vi "Test Executive.vi"(11 "Module Config":T3={"Name"="TestExec", "Parent Q"=refnum, "Is Child?"=FALSE, "Index"=0, "Dirs"={"Root"=path "", "Config"=path "C:/ATE/Config", "Logs"=path "C:/ATE/Logs", "Reports"=path "C:/ATE/Reports", "App Data"=path "C:/ProgramData/MAIN"}, "Simulate"=FALSE}) -> ()   [LabVIEW 2017]
uses:
  <vilib>/KATE/Queues/Queue Utils.lvlib
  <vilib>/KATE/Module/Module Utils.lvlib
  <vilib>/KATE/Module/Window/Window.Task, Action.ctl
  <vilib>/KATE/Event Log/Event Log.lvlib
  <vilib>/KATE/Scheduler/Scheduler.lvlib
  <vilib>/KATE/Files/File Utils.lvlib
  <vilib>/KATE/Menu/Menu Utils.lvlib
  <vilib>/KATE/Event Log/Event Log.Error Report.ctl
  <vilib>/KATE/Controls/Controls.lvlib
  Controls/TestExec.TestState.ctl
  <vilib>/KATE/Queues/Q.Element.ctl
  <vilib>/KATE/Queues/Q.Msg Return Info.ctl
  <vilib>/KATE/Queues/Q.Msg Return Data Container.ctl
  Controls/TestExec.Script Message.ctl
  <vilib>/Utility/miscctls.llb/LVRowAndColumnUnsignedTypeDef.ctl
  SubVIs/Class - ResultCntr/Class - ResultCntr.lvclass
  <vilib>/KATE/Graphics/Graphic Utils.lvlib
  <vilib>/KATE/Config/Stored Controls/Class.SaveCtrls.lvclass
  Common/TCP-IP Manager/TCP-IP Mgr.lvlib
  <vilib>/KATE/Module/Module Config.ctl
  <vilib>/KATE/Module/Module.Working Dirs.ctl
  <vilib>/KATE/Module/Module.SW Version Info.ctl
panel:
  in  "Main Tab":enum32{"Operate", "Maint"}(tab)
  out "Facility Name":string caption="Name"
  out "Error":bool
  out "Error":bool
  out "Title":string="Test Executive"
  in  "Data Tab":T1(tab)
  out "Rev":string
  in  "Sequence":u16(ring) items=["Test AAA 001", "Test BBB 002", "Test CCC 003"]
  out "Test Status Tab":enum32{"Results", "Setup"}(tab)
  out "Results":string[][](table)
  out "Setup/Instuction Figure":picture
  out "Data2DBool":bool[][](array[boolean])=[[TRUE, FALSE], [FALSE, TRUE]]
  out "Data2DStr":string[][](array[string])=[["A", "AA"], ["B", "BB"], ["C", "CC"], ["D", "DD"]]
  out "UUT State":T2={"Standby"=TRUE, "Initializing"=FALSE, "Running"=FALSE, "Error"=FALSE}
  out "Data2DFloat":dbl[][](array[numeric])
  out "Data1DFloat":dbl[](array[numeric])
  in  "ON/OFF":bool
  out "OutputY":dbl
  out "OutputX":dbl
  out "Data1DBool":bool[](array[boolean])=[TRUE, TRUE, FALSE, TRUE]
  out "Output Hist":cluster{dbl, dbl}(graph)
  in  "Equipment List":string[][](table)=[["Function Generator", "", "", "", ""], ["", "", "", "", ""], ["", "", "", "", ""], ["", "", "", "", ""], ["", "", "", "", ""]]
  out "Status":string
  out "Test Ctrl Tab":enum32{"Idle", "Running", "Completed"}(tab)
  in  "Start":bool
  out "Status Duration(s)":dbl caption="Duration(s)" format="%.1f"
  out "Status Elapsed(s)":dbl caption="Elapsed(s)" format="%.1f"
  out "Test Running":bool
  out "Progress":dbl(slide) scale=0.0..1.0
  in  "Abort":bool
  in  "Test Reset":bool
  out "Operator":string
  out "Station PN":string caption="PN"
  out "Station SN":string caption="SN"
  in  "UUT PN":string caption="PN"
  in  "UUT SN":string caption="SN"
  out "Start Time":string
  out "End Time":string
  in  "Maint":bool
  out "Logo":picture
  in  "Show Block Diagram":bool
  in  "Leave Maint":bool
  in  "SW Rev":T5={"AppName"="Test Executive", "Company"="Kwest Engineering", "Version"="0.0.3", "Description"="4/8/2017"}
  # "Facility"
  # "Station"
  # "UUT"
  # "There is a 2 sec delay from turn ON\nto Running sTATE"
  # "0"
  # "1"
  # "2"
  # "3"
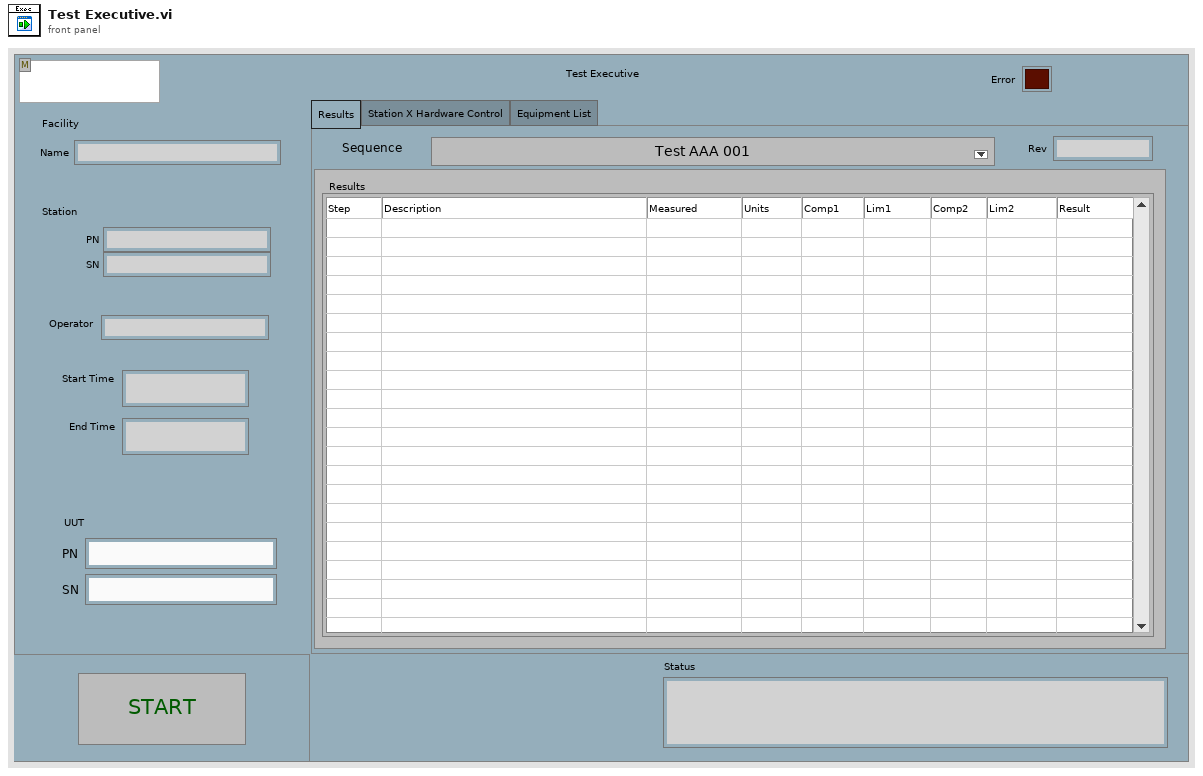
[diagram p1: front panel]
types:
  T1 = enum32{"Results", "Station X Hardware Control", "Equipment List"}
  T2 = cluster{"Standby":bool, "Initializing":bool, "Running":bool, "Error":bool}
  T3 = typedef "KATE_Lib.lvlib/Module Utils.lvlib/Module Config.ctl" = cluster{"Name":string, "Parent Q":refnum<queue>, "Is Child?":bool, "Index":i32, "Dirs":T4, "Simulate":bool}
  T4 = typedef "KATE_Lib.lvlib/Module Utils.lvlib/Module.Working Dirs.ctl" = cluster{"Root":path, "Config":path, "Logs":path, "Reports":path, "App Data":path}
  T5 = typedef "KATE_Lib.lvlib/Module Utils.lvlib/Module.SW Version Info.ctl" = cluster{"AppName":string, "Company":string, "Version":string, "Description":string}
  T6 = typedef "KATE_Lib.lvlib/Module Utils.lvlib/Module Sys Info.ctl" = cluster{"Main Q":refnum<queue>, "Exe":bool, "SW Rev":T5, "Self Ref":refnum<vi>, "Main Tab":refnum<vi>, "Pane":refnum<vi>, "Stop":cluster{"Ref":refnum<event-registration>, "Event":refnum<user-event>}, "Cfg":T3, "Services":cluster{"Name":string, "vi ref":refnum<vi>}[], "Menu Ref":refnum<k9>, "CtrlStates":refnum<class "Class.SaveCtrls.lvclass">, "Docs":cluster{"Tags":string[], "Paths":path[]}}
  T7 = enum8{"Enabled", "Disabled", "Disabled and Grayed Out"}
  T8 = typedef "LVRowAndColumnUnsignedTypeDef.ctl" = cluster{"Row":u32, "Column":u32}
  T9 = typedef "TestExec.TestState.ctl" = cluster{"Running":bool, "Results":string[][], "Start":dbl, "End":dbl, "Duration":dbl, "Failing":bool, "Abort":bool, "TC Level":i32, "TC Cnts":i32[], "Test ID":string}
  T10 = typedef "TestExec.Script Message.ctl" = cluster{"Seq":i32, "Address":string, "Function":string, "Data":variant, "Error":errorcluster}
  T11 = typedef "KATE_Lib.lvlib/Queue Utils.lvlib/Q.Msg Return Data Container.ctl" = cluster{"SeqNum":i32, "Data":variant, "Error":errorcluster}
  T12 = enum16{"Top Left", "Top Right", "Bottom Left", "Bottom Right"}
  T13 = cluster{"CtrlStates":refnum<class "Class.SaveCtrls.lvclass">, "Test":T9, "Limits":variant, "ResultID":refnum<class "Class - ResultCntr.lvclass">}
  T14 = typedef "KATE_Lib.lvlib/Queue Utils.lvlib/Q.Msg Return Info.ctl" = cluster{"Ret Q":refnum<queue>, "Ret Msg":T15, "SeqNum":i32}
  T15 = typedef "KATE_Lib.lvlib/Queue Utils.lvlib/Q.Element.ctl" = cluster{"Cmd":string, "Sub":string, "Data1":variant, "Data2":variant}
  T16 = typedef "KATE_Lib.lvlib/Event Log.lvlib/Event Log.Error Report.ctl" = cluster{"Cnt":i32, "Recent Error":errorcluster}
  T17 = typedef "KATE_Lib.lvlib/Module Utils.lvlib/Window.Task, Action.ctl" = enum16{"Resize()", "Show Panel(Bool)", "Show Scroll Bars(Bool)", "Dock to SubPanel(SubPanel Ref)", "Undock from SubPanel()", "Return to SubPanel()", "Go To Maint Tab()", "Show Maint Tab(Bool)", "Open Block Diagram()"}
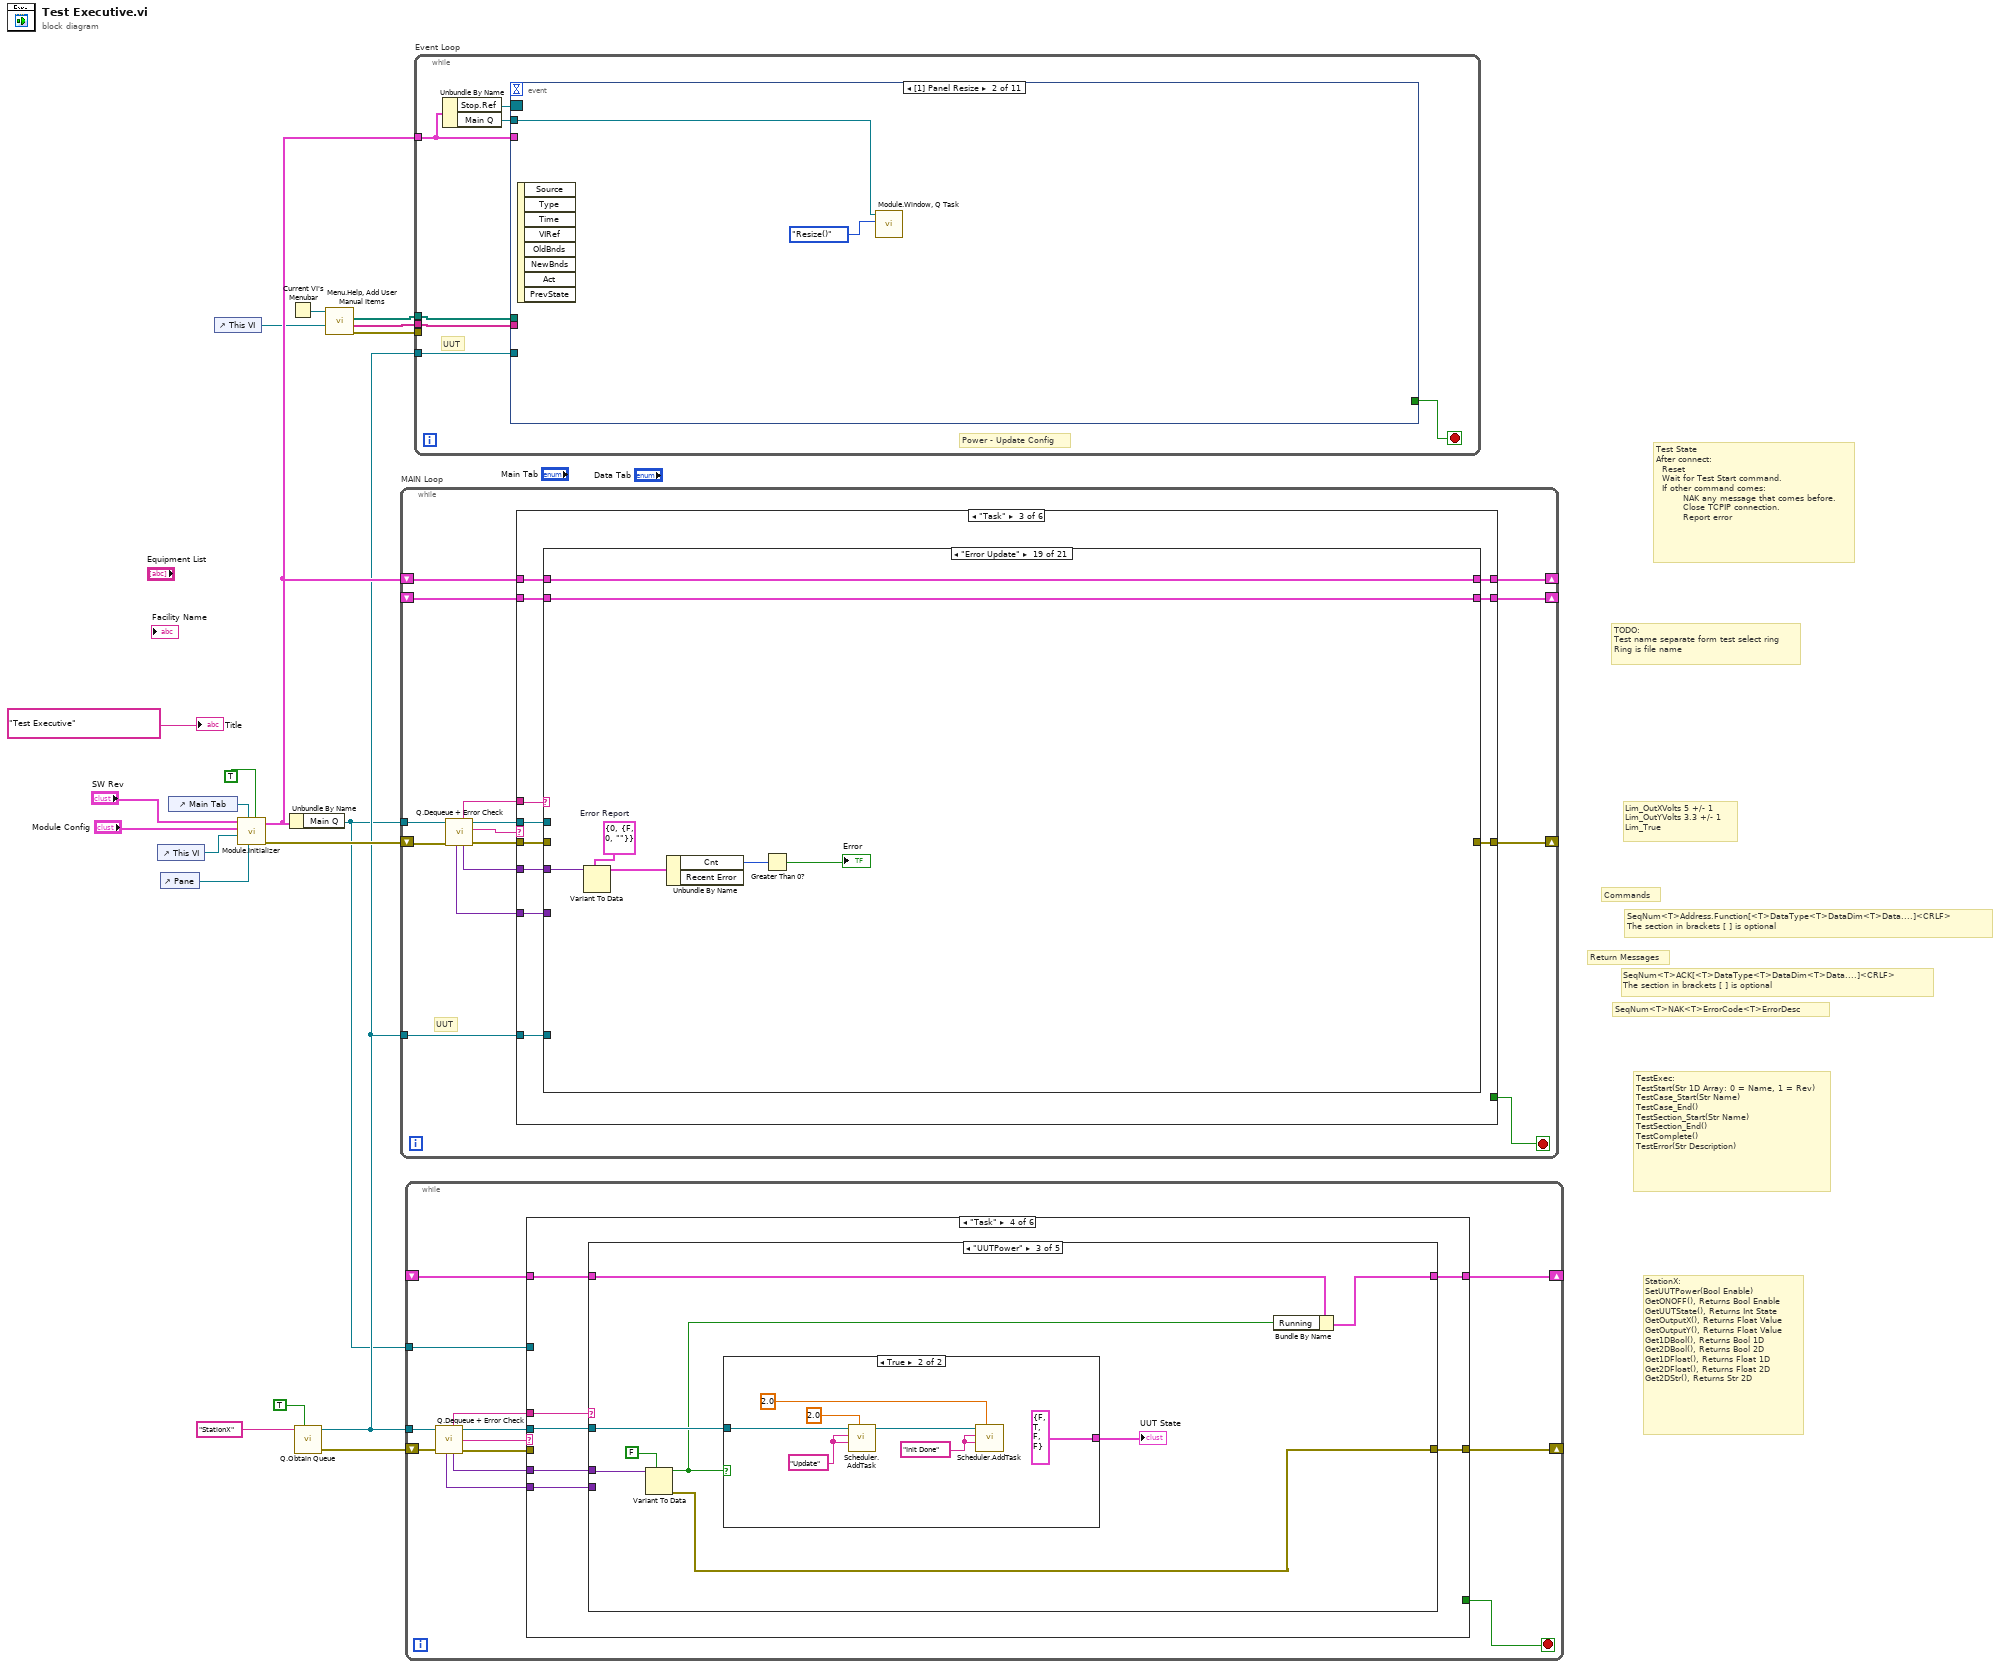
[diagram p0: block diagram]
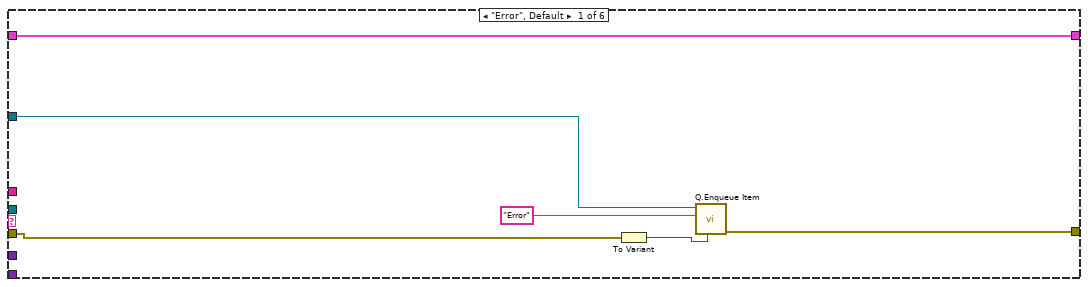
[diagram p2: hidden frame]
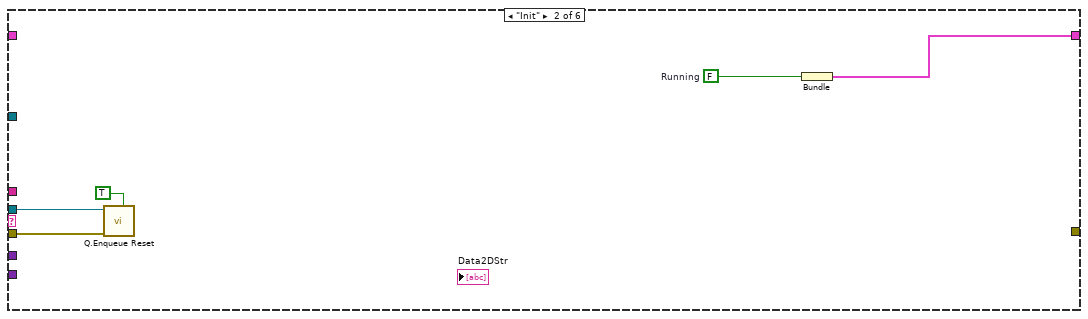
[diagram p3: hidden frame]
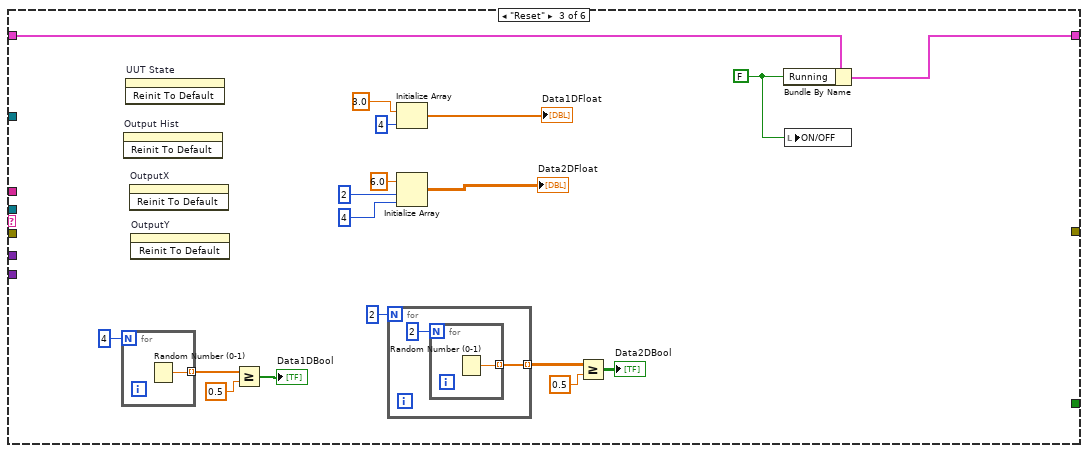
[diagram p4: hidden frame]
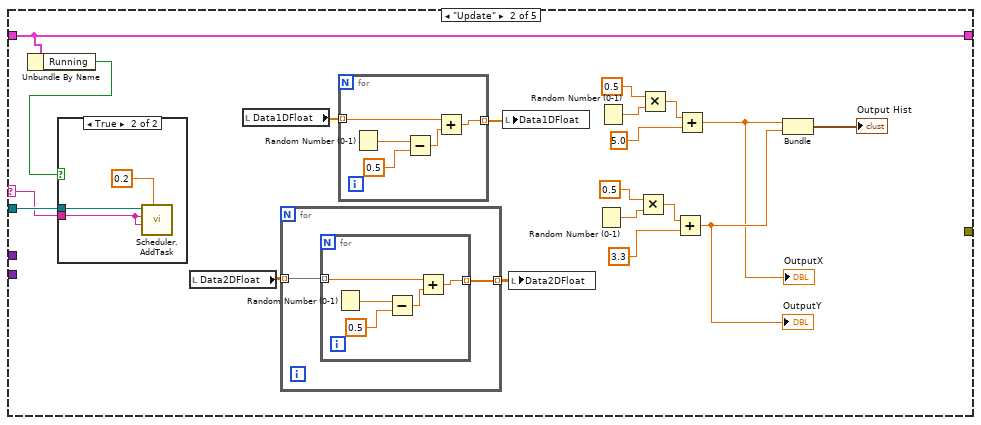
[diagram p6: hidden frame]
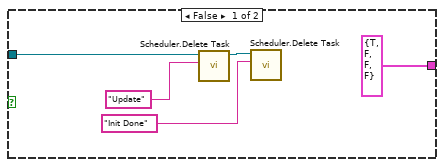
[diagram p8: hidden frame]
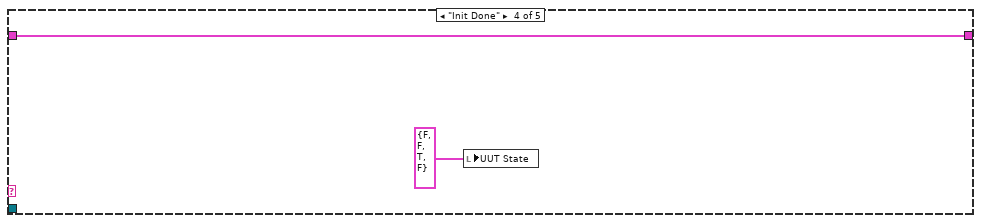
[diagram p9: hidden frame]
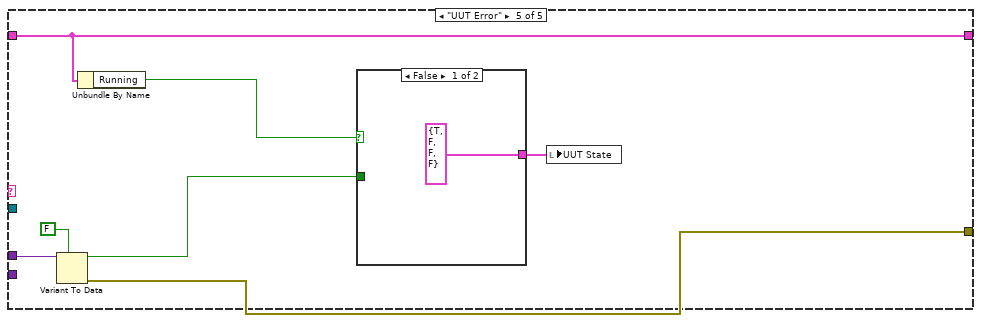
[diagram p10: hidden frame]
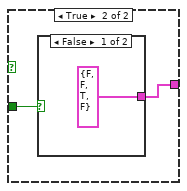
[diagram p11: hidden frame]
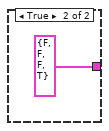
[diagram p12: hidden frame]
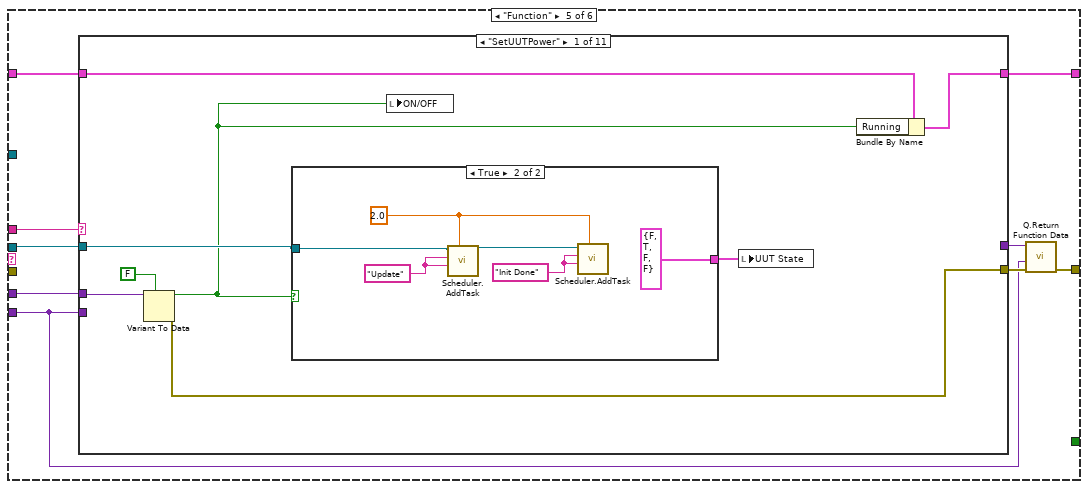
[diagram p13: hidden frame]
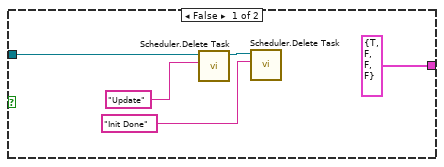
[diagram p14: hidden frame]
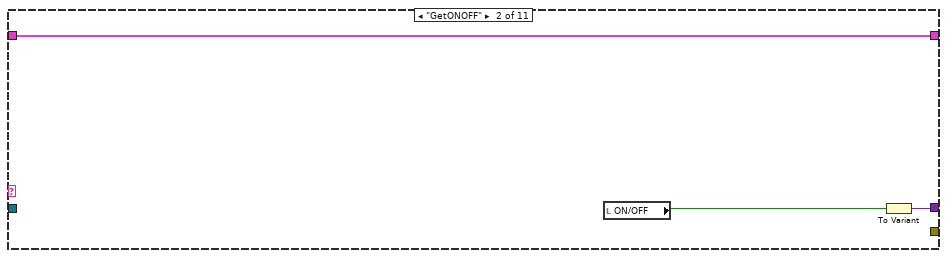
[diagram p15: hidden frame]
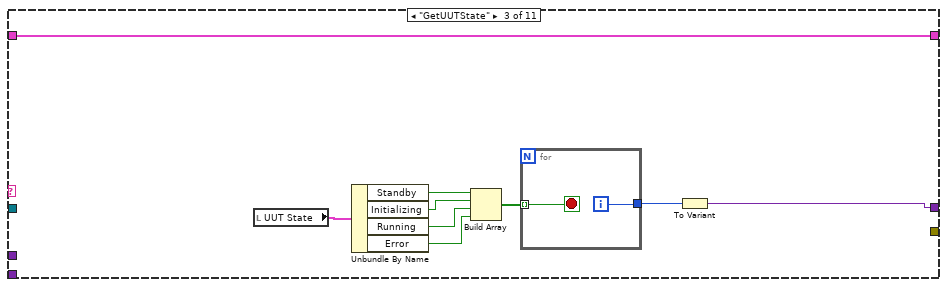
[diagram p16: hidden frame]
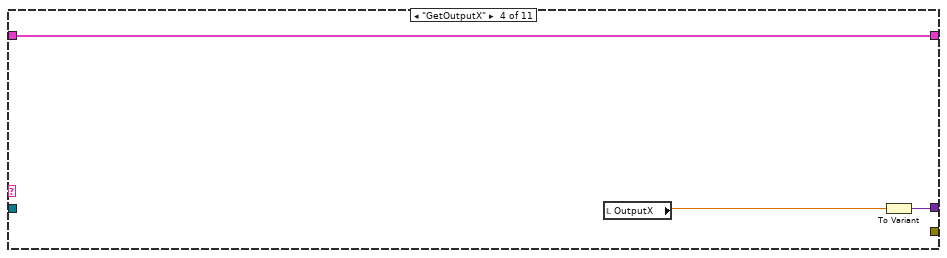
[diagram p17: hidden frame]
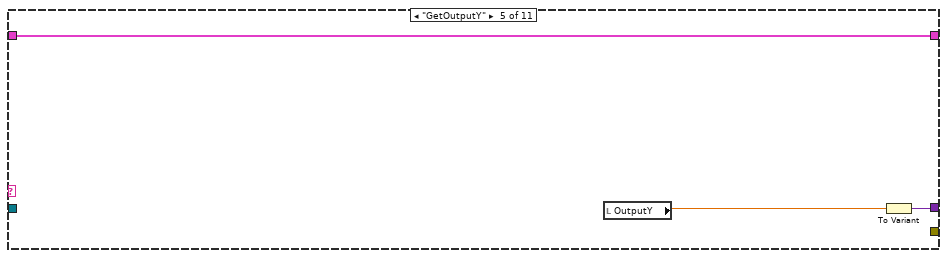
[diagram p18: hidden frame]
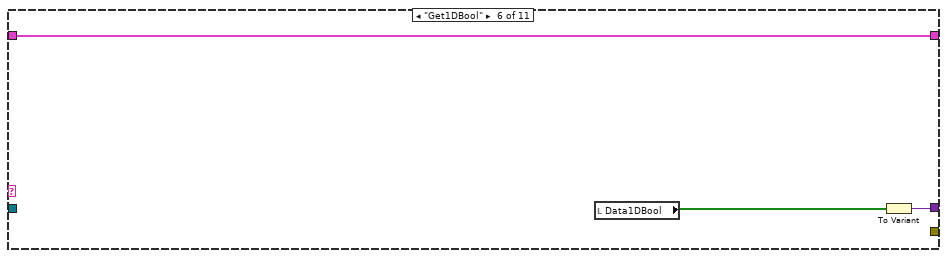
[diagram p19: hidden frame]
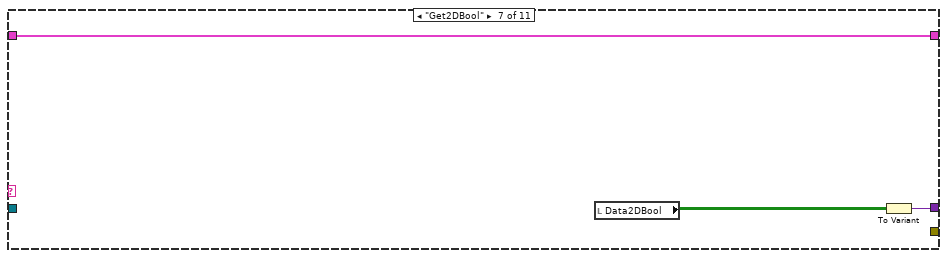
[diagram p20: hidden frame]
diagram:
  # "TODO:\nTest name separate form test select ring\nRing is file name"
  # "Test State\nAfter connect:\n  Reset\n  Wait for Test Start command.\n  If other command comes: \n         NAK any message that comes before.\n         Close TCPIP connection.\n         Report error"
  # "Lim_OutXVolts 5 +/- 1\nLim_OutYVolts 3.3 +/- 1\nLim_True"
  # "Return Messages"
  # "Commands"
  # "SeqNum<T>NAK<T>ErrorCode<T>ErrorDesc"
  # "SeqNum<T>ACK[<T>DataType<T>DataDim<T>Data....]<CRLF>  \nThe section in brackets [ ] is optional"
  # "SeqNum<T>Address.Function[<T>DataType<T>DataDim<T>Data....]<CRLF>\nThe section in brackets [ ] is optional"
  # "StationX:\nSetUUTPower(Bool Enable)\nGetONOFF(), Returns Bool Enable\nGetUUTState(), Returns Int State\nGetOutputX(), Returns Float Value\nGetOutputY(), Returns Float Value\nGet1DBool(), Returns Bool 1D\nGet2DBool(), Returns Bool 2D\nGet1DFloat(), Returns Float 1D\nGet2DFloat(), Returns Float 2D\nGet2DStr(), Returns Str 2D"
  # "TestExec:\nTestStart(Str 1D Array: 0 = Name, 1 = Rev)\nTestCase_Start(Str Name)\nTestCase_End()\nTestSection_Start(Str Name)\nTestSection_End()\nTestComplete()\nTestError(Str Description)"
  n1 = control-ref of="This VI"() -> (w17:refnum<vi>)
  n2 = control-ref of="Pane"() -> (w16:refnum<vi>)
  n3 = control-ref of="Main Tab"() -> (w18:refnum<vi>)
  n4 = control-ref of="This VI"() -> (w3:refnum<vi>)
  n5 = call <vilib>:"Module.Initializer.vi"("Menu Ref"=TRUE ("En Event Log"), "Pane"=w16, "Main Tab"=w18, "Self Ref"=w17, "Module Config"="Module Config", "SW Rev"="SW Rev") -> ("error out"=w19:errorcluster, "Sys"=w9:T6)  [unwired: 4 in]
  n6 = Current VI's Menubar() -> (w13:refnum<k9>)
  n7 = Unbundle By Name(w9) -> ("Main Q"=w4:refnum<queue>)
  n8 = call <vilib>:"Q.Obtain Queue.vi"("Enqueue Init"=TRUE, "Q Name"="StationX" ("Name")) -> ("error out"=w8:errorcluster, "Q Out"=w5:refnum<queue>)  [unwired: 7 in, 1 out]
  n9 = call <vilib>:"Menu.Help, Add User Manual Items.vi"("Main VI"=w3, "Menu Ref"=w13) -> ("error out"=w12:errorcluster, "Tags"=w11:string[], "Paths"=w10:path[])  [unwired: 6 in, 1 out]
  n10 = while "MAIN Loop" {
    shift-right: [w30] -> _
    shift-left: w19 -> [w28]
    shift-right: [w31] -> _
    shift-left: _ -> [w34]
    shift-right: [w32] -> _
    shift-left: w9 -> [w33]
    tunnel: w4 -> [w27]
    tunnel: w5 -> [w20]
    stop <- w21 stop-if-true
    # "UUT"
    n11 = call <vilib>:"Q.Dequeue + Error Check.vi"("Error In"=w28, "Q In"=w27) -> ("error out"=w29:errorcluster, "Cmd"=w26:string, "Q Out"=w25:refnum<queue>, "Data1"=w24:variant, "Sub"=w22:string, "Data2"=w23:variant)  [unwired: 4 in]
    n12 = case shown="\"Task\"" w26 {
      selector: w26 -> [_ _ _ _ w668 _]
      tunnel: w34 -> [_ w87 w135 w531 w662 w715]
      tunnel: w33 -> [w42 w117 w136 w532 w670 w716]
      tunnel: [w42 w117 w134 w530 w670 w716] -> w32
      tunnel: [w39 w120 w133 w529 w661 w715] -> w31
      tunnel: [w36 _ w127 w524 w669 w718] -> w30
      tunnel: w29 -> [w44 w124 w129 w525 w666 _]
      tunnel: w25 -> [w45 w125 w130 w526 w664 _]
      tunnel: w24 -> [_ _ w131 w527 w667 _]
      tunnel: w23 -> [_ _ w128 w523 _ _]
      tunnel: w22 -> [_ _ w132 w528 w665 _]
      tunnel: [_ _ _ _ _ TRUE] -> w21
      tunnel: w20 -> [_ _ w126 _ _ w712]
      frame "Init" {
        n13 = call <vilib>:"Q.Enqueue Reset.vi"("Top of Q(T)"=FALSE ("Flush Q"), "Error In"=w44, "Q In"=w45) -> ("Q Out"=w35:refnum<queue>)  [unwired: 7 in, 1 out]
        n14 = stacked-sequence {
          tunnel: w42 -> [w49 w61 _ w83]
          tunnel: [_ w62 _ _] -> w41
          tunnel: [_ _ w79 _] -> w40
          tunnel: [_ _ w78 _] -> w38
          tunnel: [_ _ w77 _] -> w37
          tunnel: w35 -> [_ _ _ w84]
          tunnel: [_ _ _ w80] -> w36
          frame #0 {
            # "Only allow \"Show block diagram\" in development"
            n15 = call <vilib>:"Application Directory.vi"() -> ("Application Directory"=w48:path)
            n16 = Unbundle By Name(w49) -> ()  [unwired: 1 out]
            n17 = Build Path(base path=w48, name or relative path="Company Logo.png") -> (appended path=w46:path)
            n18 = Unbundle By Name(w49) -> ("Exe"=w56:bool)
            n19 = call <vilib>:"Image File to 2D Image.vi"("Path"=w46) -> ("2D Picture"=→"Logo":picture)  [unwired: 9 in, 1 out]
            n20 = Not(x=w56) -> (.not. x?=w57:bool)
            n21 = property on="Show Block Diagram" class="Bool"("Visible"=w57) -> ()  [unwired: 2 in, 2 out]
            n22 = property class="App"() -> ("App.UserName"=→"Operator":string)  [unwired: 2 in, 2 out]
            n23 = call <vilib>:"Event Log.Record Event.vi"("Message"="Application Launched") -> ()  [unwired: 10 in, 1 out]
            "Test Status Tab" <- enum32{"Results", "Setup"}."Results" ("Test Status Tab")
            "Station PN" <- "TS1034" ("Station PN")
            "Station SN" <- "001" ("Station PN")
          }
          frame #1 {
            (unwired) refnum<vi>[] []
            # "Restore saved control states"
            n24 = Unbundle By Name(w61) -> ("Cfg.Name"=w60:string, "Cfg.Dirs.App Data"=w59:path)
            n25 = while {
              shift-right: [w65] -> w58
              shift-left: _ -> [w66]
              i -> [w67]
              stop <- w64 stop-if-true
              n26 = case shown="0" w67 {
                tunnel: w66 -> [w69 w75]
                tunnel: [w69 w76] -> w65
                tunnel: [TRUE _] -> w64
                frame Default {
                  # "Done"
                }
                frame 0 {
                  w71 = refnum<vi> refnum  # Control
                  n27 = control-ref of="Sequence"() -> (w73:refnum<vi>)
                  n28 = control-ref of="Equipment List"() -> (w72:refnum<vi>)
                  n29 = To More Generic Class(target class=w71, reference=w73) -> (generic class reference=w74:refnum<vi>)
                  n30 = To More Generic Class(target class=w71, reference=w72) -> (generic class reference=w70:refnum<vi>)
                  n31 = Build Array (concatenate)(w75, w74, w70) -> (w76:refnum<vi>[])
                }
              }
            }
            n32 = call-dynamic "Class.SaveCtrls.InitLoadRestore.vi"("Ctrl Array"=w58, "Module Data Dir"=w59, "Module Name"=w60, "CtrlStates In"=refnum<class "Class.SaveCtrls.lvclass"> refnum) -> ("CtrlStates"=w62:refnum<class "Class.SaveCtrls.lvclass">)  [unwired: 6 in, 1 out]
          }
          frame #2 {
            w77 = refnum<class "Class - ResultCntr.lvclass"> refnum  # ResultID
            w78 = variant  # Limits
            w79 = T9 {"Running"=FALSE, "Results"=[], "Start"=0.0, "End"=0.0, "Duration"=0.0, "Failing"=FALSE, "Abort"=FALSE, "TC Level"=0, "TC Cnts"=[], "Test ID"=""}  # Test
          }
          frame #3 {
            # "Launch TCP-IP Listener"
            n33 = Unbundle By Name(w83) -> ("Cfg.Dirs"=w82:T4)
            n34 = call "TCP-IP Mgr.Create.vi"("Working Dirs"=w82, "Q In"=w84) -> ("Error Out"=w81:errorcluster)  [unwired: 7 in, 2 out]
            n35 = call "TCP-IP Mgr.Show.vi"("error in"=w81) -> ("error out"=w80:errorcluster)  [unwired: 10 in]
          }
        }
        n36 = Bundle("CtrlStates"=w41, "Test"=w40, "Limits"=w38, "ResultID"=w37) -> (w39:T13)  [unwired: 1 in]
      }
      frame "Reset" {
        w91 = FALSE ("Error")
        w105 = 0.0 ("Elapsed(s)")
        w107 = T9 {"Running"=FALSE, "Results"=[], "Start"=0.0, "End"=0.0, "Duration"=0.0, "Failing"=FALSE, "Abort"=FALSE, "TC Level"=0, "TC Cnts"=[], "Test ID"=""}  # Test
        w121 = 0
        n37 = call <vilib>:"Scheduler.Clear-Reset.vi"("error in"=w124, "Q In"=w125) -> ("error out"=w108:errorcluster, "Q Out"=w109:refnum<queue>)  [unwired: 8 in]
        n38 = Current VI's Menubar() -> (w112:refnum<k9>)
        n39 = property on="Error" class="Bool (strict)"("Visible"=FALSE) -> ()  [unwired: 2 in, 2 out]
        n40 = invoke on="Progress" class="Slide (strict)" method="Reinit To Default"() -> ()  [unwired: 3 in, 3 out]
        n41 = call <vilib>:"Menu.Enable Item.vi"("Enable"=TRUE, "Tag"="Config", "Menu Ref"=w112) -> ()  [unwired: 7 in, 2 out]
        n42 = invoke on="Error" class="Bool (strict)" method="Reinit To Default"() -> ()  [unwired: 3 in, 3 out]
        n43 = To Variant(anything=FALSE) -> (Variant=w115:variant)
        n44 = property on="Sequence" class="Ring (strict)"("Strings []"=string[] ["Test AAA 001", "Test BBB 002", "Test CCC 003"]) -> ()  [unwired: 2 in, 2 out]
        n45 = call <vilib>:"Q.Enqueue Task.vi"("Data1"=w115, "Error In"=w108, "Task Name"="Lock Test Controls", "Q In"=w109) -> ("error out"=w100:errorcluster, "Q Out"=w101:refnum<queue>)  [unwired: 6 in]
        n46 = call <vilib>:"Q.Enqueue Task.vi"("Error In"=w100, "Task Name"="Init Limits", "Q In"=w101) -> ("error out"=w97:errorcluster, "Q Out"=w98:refnum<queue>)  [unwired: 7 in]
        n47 = call <vilib>:"Q.Enqueue Task.vi"("Error In"=w97, "Task Name"="TCP_IP Clear Log", "Q In"=w98) -> ("error out"=w95:errorcluster, "Q Out"=w96:refnum<queue>)  [unwired: 7 in]
        n48 = Unbundle By Name(w87) -> ("ResultID"=w88:refnum<class "Class - ResultCntr.lvclass">)
        n49 = call <vilib>:"Q.Enqueue Task.vi"("Error In"=w95, "Task Name"="Initialization Done", "Q In"=w96) -> ()  [unwired: 7 in, 2 out]
        n50 = call "Class - ResultCntr.Init.vi"("Class - ResultCntr in"=w88) -> ("Class - ResultCntr out"=w85:refnum<class "Class - ResultCntr.lvclass">)  [unwired: 9 in, 1 out]
        n51 = Bundle By Name(cluster=w87, "ResultID"=w85) -> (w86:T13)
        n52 = property on="Error" class="Bool (strict)"("Value"=w91, "Visible"=w91, "TipStrip"="" ("Tip Strip")) -> ()  [unwired: 2 in, 2 out]
        n53 = local write "Main Tab"(w121) -> ()
        n54 = local write "Data Tab"(w121) -> ()
        n55 = local write "Test Ctrl Tab"(enum32{"Idle", "Running", "Completed"}."Idle" ("Test Ctrl Tab")) -> ()
        n56 = local write "Status"("Initializing" ("Status")) -> ()
        n57 = call <vilib>:"Event Log.Record Event.vi"("Message"="Initialized") -> ()  [unwired: 10 in, 1 out]
        n58 = property on="Start" class="Bool"("DisabledEnum"=T7."Disabled and Grayed Out" ("Disabled")) -> ()  [unwired: 2 in, 2 out]
        n59 = invoke on="Start Time" class="Str" method="Reinit To Default"() -> ()  [unwired: 3 in, 3 out]
        n60 = invoke on="End Time" class="Str" method="Reinit To Default"() -> ()  [unwired: 3 in, 3 out]
        n61 = invoke on="Results" class="Tbl (strict)" method="Reinit To Default"() -> ()  [unwired: 3 in, 3 out]
        n62 = Initialize Array(0, 10) -> (w102:i32[])
        n63 = invoke on="UUT PN" class="Str" method="Reinit To Default"() -> ()  [unwired: 3 in, 3 out]
        n64 = invoke on="UUT SN" class="Str" method="Reinit To Default"() -> ()  [unwired: 3 in, 3 out]
        n65 = property on="Status" class="Str"("Text.BGColor"=u32 13816530) -> ()  [unwired: 2 in, 2 out]
        n66 = Bundle By Name(cluster=w86, "Test"=w107, "Test.TC Cnts"=w102) -> (w120:T13)
        n67 = invoke on="Rev" class="Str" method="Reinit To Default"() -> ()  [unwired: 3 in, 3 out]
        "Status Elapsed(s)" <- w105
        "Status Duration(s)" <- w105
        "Start Time" <- "" ("Start Time")
      }
      frame "Task" {
        n68 = case shown="\"Error Update\"" w132 {
          selector: w132 -> [_ _ _ w162 _ _ _ w296 _ _ _ _ _ _ _ _ _ _ _ _ w518]
          tunnel: w136 -> [w143 w152 w157 w166 w240 w269 w289 w303 w325 w341 w357 w368 w391 w400 w408 w452 w459 w482 w489 w492 w519]
          tunnel: w135 -> [w142 w151 w156 w159 w239 w242 w287 w291 w313 w333 w349 w360 w378 w396 w411 w451 w456 w481 w488 w493 w520]
          tunnel: [w143 w152 w157 w166 w240 w269 w289 w303 w325 w341 w357 w368 w391 w400 w408 w452 w459 w482 w489 w492 w519] -> w134
          tunnel: [w142 w151 w156 w159 w239 w253 w286 w291 w312 w332 w348 w359 w387 w395 w411 w451 w456 w481 w488 w493 w520] -> w133
          tunnel: w131 -> [w141 _ _ w165 _ w260 w283 _ w318 w331 w347 _ _ _ w410 w450 w458 w476 w487 _ w517]
          tunnel: w130 -> [_ _ _ w161 w238 w250 _ w301 w320 w336 w352 w363 w389 _ w402 _ w453 w479 _ _ _]
          tunnel: w129 -> [_ _ _ _ _ _ _ _ _ _ _ _ _ _ _ _ _ _ _ _ w515]
          tunnel: w128 -> [_ _ _ _ _ _ _ _ _ _ _ _ _ _ _ _ _ w477 _ _ w516]
          tunnel: [w137 _ _ _ _ w259 _ _ w315 w326 w342 _ _ _ w403 w447 _ w469 _ _ w514] -> w127
          tunnel: w126 -> [_ _ _ _ _ _ _ _ _ _ _ _ w370 w393 w407 _ _ _ _ _ _]
          frame "Lock Test Controls" {
            n69 = Variant To Data(type=FALSE, Variant=w141) -> (data=w138:bool, error out=w139:errorcluster)  [unwired: 1 in]
            n70 = case shown="No Error" w139 {
              selector: w139 -> [_ w150]
              tunnel: w138 -> [w145 _]
              tunnel: [_ w150] -> w137
              frame No Error {
                n71 = case shown="False" w145 {
                  tunnel: [T7."Enabled" ("Disabled") T7."Disabled and Grayed Out" ("Disabled")] -> w144
                  tunnel: [T7."Enabled" ("Disabled") T7."Disabled" ("Disabled")] -> _
                  frame False {
                  }
                  frame True {
                  }
                }
                n72 = property on="UUT PN" class="Str"("DisabledEnum"=w144) -> ()  [unwired: 2 in, 2 out]
                n73 = property on="Sequence" class="Ring (strict)"("DisabledEnum"=w144) -> ()  [unwired: 2 in, 2 out]
                n74 = property on="UUT SN" class="Str"("DisabledEnum"=w144) -> ()  [unwired: 2 in, 2 out]
              }
              frame Error {
              }
            }
          }
          frame "Init Limits" {
          }
          frame "Initialization Done" {
            n75 = property on="Status" class="Str"("Text.BGColor"=u32 13816530) -> ()  [unwired: 2 in, 2 out]
            n76 = property on="Start" class="Bool"("DisabledEnum"=T7."Enabled" ("Disabled")) -> ()  [unwired: 2 in, 2 out]
            "Status" <- "Ready" ("Status")
          }
          frame "Simulate Test Seq" {
            n77 = Unbundle By Name(w159) -> ("Test.Running"=w158:bool)
            n78 = Variant To Data(type=0, Variant=w165) -> (data=w163:i32)  [unwired: 1 in, 1 out]
            n79 = case shown="True" w158 {
              tunnel: w163 -> [_ w170]
              tunnel: w162 -> [_ w173]
              tunnel: w161 -> [_ w174]
              tunnel: 0.2 ("Interval(s)") -> [_ w171]
              frame False {
              }
              frame True {
                n80 = Increment(x=w170) -> (x+1=w172:i32)
                n81 = call <vilib>:"Scheduler.AddTask.vi"("Data1"=w172, "Interval(s)"=w171, "Task Name"=w173, "Sched Name"=w173, "Q In"=w174) -> ("Q Out"=w169:refnum<queue>)  [unwired: 5 in, 1 out]
                n82 = case shown="2" w170 {
                  tunnel: [w176 w181 w184 w187 w190 w193 w196 _ w200 w203 w206 w209 w212 w215 _ w219 w222 w225 _ _] -> w168
                  tunnel: ["Test Start" "TestCase_Start" "Result" "Result" "TestSection_Start" "Result" "Result" "TestSection_End" "Result" "Result" "TestCase_Start" "TestSection_Start" "Result" "Result" "TestSection_End" "TestSection_Start" "Result" "Result" "TestSection_End" "Test Complete"] -> w167
                  frame 0, Default {
                    n83 = Build Array("Sim Test AABBCC", "V0.1.3") -> (w177:string[])
                    n84 = To Variant(anything=w177) -> (Variant=w176:variant)
                  }
                  frame 1 {
                    n85 = To Variant(anything="Test Case AAA") -> (Variant=w181:variant)
                  }
                  frame 2 {
                    n86 = To Variant(anything=string[] ["Output X Voltage", "5", "Lim_OutXVolts"]) -> (Variant=w184:variant)
                  }
                  frame 3 {
                    n87 = To Variant(anything=string[] ["Output Y Voltage", "3.3", "Lim_OutYVolts"]) -> (Variant=w187:variant)
                  }
                  frame 4 {
                    n88 = To Variant(anything="Test Section XX") -> (Variant=w190:variant)
                  }
                  frame 5 {
                    n89 = To Variant(anything=string[] ["Output X Voltage", "5", "Lim_OutXVolts"]) -> (Variant=w193:variant)
                  }
                  frame 6 {
                    n90 = To Variant(anything=string[] ["Output Y Voltage", "3.3", "Lim_OutYVolts"]) -> (Variant=w196:variant)
                  }
                  frame 7 {
                  }
                  frame 8 {
                    n91 = To Variant(anything=string[] ["Output X Voltage", "5", "Lim_OutXVolts"]) -> (Variant=w200:variant)
                  }
                  frame 9 {
                    n92 = To Variant(anything=string[] ["Output Y Voltage", "3.3", "Lim_OutYVolts"]) -> (Variant=w203:variant)
                  }
                  frame 10 {
                    n93 = To Variant(anything="Test Case BB") -> (Variant=w206:variant)
                  }
                  frame 11 {
                    n94 = To Variant(anything="Test Section YY") -> (Variant=w209:variant)
                  }
                  frame 12 {
                    n95 = To Variant(anything=string[] ["Output X Voltage", "5", "Lim_OutXVolts"]) -> (Variant=w212:variant)
                  }
                  frame 13 {
                    n96 = To Variant(anything=string[] ["Output Y Voltage", "3.3", "Lim_OutYVolts"]) -> (Variant=w215:variant)
                  }
                  frame 14 {
                  }
                  frame 15 {
                    n97 = To Variant(anything="Test Section YY") -> (Variant=w219:variant)
                  }
                  frame 16 {
                    n98 = To Variant(anything=string[] ["Output X Voltage", "5", "Lim_OutXVolts"]) -> (Variant=w222:variant)
                  }
                  frame 17 {
                    n99 = To Variant(anything=string[] ["Output Y Voltage", "3.3", "Lim_OutYVolts"]) -> (Variant=w225:variant)
                  }
                  frame 18 {
                  }
                  frame 19 {
                  }
                }
                n100 = call <vilib>:"Q.Enqueue Task.vi"("Data1"=w168, "Task Name"=w167, "Q In"=w169) -> ()  [unwired: 7 in, 2 out]
              }
            }
          }
          frame "Launch Test Script" {
            # "TODO: Launch Script\nFor now, run simulation"
            n101 = property on="Sequence" class="Ring (strict)"() -> ("Strings []"=w233:string[])  [unwired: 2 in, 2 out]
            n102 = Index Array(array=w233, index="Sequence") -> (element=w232:string)
            n103 = property on="Sequence" class="Ring (strict)"("RingText.Text"=w232) -> ()  [unwired: 2 in, 2 out]
            n104 = Build Array(w232, "1.0.2" ("Task Name")) -> (w235:string[])
            n105 = call <vilib>:"Q.Enqueue Task.vi"("Data1"=w235, "Task Name"="Test Start", "Q In"=w238) -> ("Q Out"=w231:refnum<queue>)  [unwired: 7 in, 1 out]
            n106 = call <vilib>:"Q.Enqueue Task.vi"("Data1"=0, "Task Name"="Simulate Test Seq", "Q In"=w231) -> ()  [unwired: 7 in, 2 out]
          }
          frame "Test Start" {
            w261 = 0.0 ("Elapsed(s)")
            # "TODO: Kill timeout for the script start"
            n107 = Variant To Data(type=string[] [], Variant=w260) -> (data=w257:string[], error out=w259:errorcluster)  [unwired: 1 in]
            n108 = Current VI's Menubar() -> (w266:refnum<k9>)
            n109 = call <vilib>:"Menu.Enable Item.vi"("Enable"=FALSE, "Tag"="Config", "Menu Ref"=w266) -> ()  [unwired: 7 in, 2 out]
            n110 = call <vilib>:"Q.Enqueue Task.vi"("Task Name"="Test Status", "Q In"=w250) -> ()  [unwired: 8 in, 2 out]
            n111 = Index Array(array=w257) -> (element #1=w255:string, element #2=w254:string)  [unwired: 2 in]
            "Rev" <- w254
            n112 = Unbundle By Name(w242) -> ("ResultID"=w244:refnum<class "Class - ResultCntr.lvclass">)
            n113 = call "Class - ResultCntr.Init.vi"("Class - ResultCntr in"=w244) -> ("Class - ResultCntr out"=w241:refnum<class "Class - ResultCntr.lvclass">)  [unwired: 9 in, 1 out]
            n114 = Bundle By Name(cluster=w242, "ResultID"=w241) -> (w243:T13)
            n115 = property on="Sequence" class="Ring (strict)"("RingText.Text"=w255) -> ()  [unwired: 2 in, 2 out]
            n116 = invoke on="Results" class="Tbl (strict)" method="Reinit To Default"() -> ()  [unwired: 3 in, 3 out]
            n117 = property on="Results" class="Tbl (strict)"("Index Values"=T8 {"Row"=0, "Column"=0}) -> ()  [unwired: 2 in, 2 out]
            n118 = Concatenate Strings("Test Sequence Start: " ("Message"), w255, ", Rev ", w254) -> (w263:string)
            n119 = Format Date/Time String() -> (date/time string=w262:string)  [unwired: 3 in]
            n120 = call <vilib>:"High Resolution Relative Seconds.vi"() -> ("relative seconds"=w251:dbl)
            n121 = local write "Start Time"(w262) -> ()
            n122 = local write "Status"(w263) -> ()
            n123 = call <vilib>:"Event Log.Record Event.vi"("Message"=w263) -> ()  [unwired: 10 in, 1 out]
            n124 = Bundle By Name(cluster=w243, "Test.Running"=TRUE, "Test.Start"=w251, "Test.Duration"=60.0, "Test.TC Level"=0, "Test.TC Cnts"=i32[] [0, 0, 0, 0, 0, 0, 0, 0, 0, 0]) -> (w253:T13)
            n125 = local write "Status Duration(s)"(w261) -> ()
            n126 = local write "Status Elapsed(s)"(w261) -> ()
            n127 = local write "Test Ctrl Tab"(1) -> ()
          }
          frame "Result" {
            # "Skip Limit Name"
            # "Unpack Result Data Type\nEvaluate PASS/FAIL\nSave Result"
            n128 = Variant To Data(type=string[] [], Variant=w283) -> (data=w281:string[])  [unwired: 1 in, 1 out]
            n129 = Unbundle By Name(w287) -> ("ResultID"=w272:refnum<class "Class - ResultCntr.lvclass">)
            n130 = Index Array(array=w281) -> (element #1=w280:string, element #2=w279:string, element #3=w278:string, element #5=w276:string, element #6=w275:string, element #7=w274:string, element #8=w273:string)  [unwired: 8 in, 1 out]
            n131 = call "Class - ResultCntr.AddResultID.vi"("Class - ResultCntr in"=w272) -> ("ID"=w270:string, "Class - ResultCntr out"=w271:refnum<class "Class - ResultCntr.lvclass">)  [unwired: 8 in, 1 out]
            n132 = local read "Results"() -> (w288:string[][])
            n133 = Build Array(w270, w280, w279, w278, w276, w275, w274, w273, "PASS") -> (w285:string[])
            n134 = Bundle By Name(cluster=w287, "ResultID"=w271, "Test.Test ID"=w270) -> (w286:T13)
            n135 = Build Array (concatenate)(w288, w285) -> (w284:string[][])
            n136 = local write "Results"(w284) -> ()
          }
          frame "Test Status" {
            w294 = 1.0 ("y")
            # "Dur"
            # "Elapsed"
            n137 = Unbundle By Name(w291) -> ("Test.Start"=w298:dbl, "Test.Duration"=w297:dbl)
            n138 = call <vilib>:"High Resolution Relative Seconds.vi"() -> ("relative seconds"=w302:dbl)
            n139 = Subtract(x=w302, y=w298) -> (x-y=w299:dbl)
            n140 = Subtract(x=w299, y=w297) -> (x-y=w300:dbl)
            n141 = Divide(x=w299, y=w297) -> (x/y=w292:dbl)
            n142 = Greater Or Equal?(x=w292, y=w294) -> (x >= y?=w293:bool)
            n143 = Unbundle By Name(w291) -> ("Test.Running"=w290:bool)
            n144 = Select(t=w294, s=w293, f=w292) -> (s? t:f=w295:dbl)
            n145 = local write "Status Elapsed(s)"(w299) -> ()
            n146 = local write "Progress"(w295) -> ()
            n147 = case shown="True" w290 {
              tunnel: w301 -> [w305 w311]
              tunnel: w300 -> [_ w308]
              tunnel: w296 -> [_ w306]
              frame False {
                w304 = "Test Complete"
                n148 = call <vilib>:"Q.Enqueue Task.vi"("Task Name"=w304, "Q In"=w305) -> ()  [unwired: 8 in, 2 out]
                n149 = local write "Status"(w304) -> ()
              }
              frame True {
                w309 = 0.1 ("Interval(s)")
                n150 = Greater?(x=w308, y=w309) -> (0:w310:bool)
                n151 = Select(t=w309, s=w310, f=w308) -> (s? t:f=w307:dbl)
                n152 = call <vilib>:"Scheduler.AddTask.vi"("Interval(s)"=w307, "Task Name"=w306, "Sched Name"=w306, "Q In"=w311) -> ()  [unwired: 6 in, 2 out]
              }
            }
          }
          frame "Test Abort" {
            n153 = Variant To Data(type="", Variant=w318) -> (data=w316:string, error out=w315:errorcluster)  [unwired: 1 in]
            n154 = call <vilib>:"Scheduler.Clear-Reset.vi"("Q In"=w320) -> ("error out"=w322:errorcluster, "Q Out"=w323:refnum<queue>)  [unwired: 9 in]
            n155 = Flush Queue(queue=w323, error in (no error)=w322) -> (queue out=w324:refnum<queue>)  [unwired: 2 out]
            n156 = call <vilib>:"Q.Enqueue Task.vi"("Task Name"="Test Complete", "Q In"=w324) -> ()  [unwired: 8 in, 2 out]
            n157 = call <vilib>:"Event Log.Record Event.vi"("Message"=w316) -> ()  [unwired: 10 in, 1 out]
            n158 = local write "Status"(w316) -> ()
            n159 = property on="Status" class="Str"("Text.BGColor"=u32 16757760) -> ()  [unwired: 2 in, 2 out]
            n160 = Bundle By Name(cluster=w313, "Test.Running"=FALSE) -> (w312:T13)
          }
          frame "Test Fail" {
            n161 = Variant To Data(type="", Variant=w331) -> (data=w328:string, error out=w326:errorcluster)  [unwired: 1 in]
            n162 = call <vilib>:"Scheduler.Clear-Reset.vi"("Q In"=w336) -> ("error out"=w338:errorcluster, "Q Out"=w339:refnum<queue>)  [unwired: 9 in]
            n163 = Flush Queue(queue=w339, error in (no error)=w338) -> (queue out=w340:refnum<queue>)  [unwired: 2 out]
            n164 = Concatenate Strings("Test FAIL!!\n", w328) -> (w327:string)
            n165 = call <vilib>:"Q.Enqueue Task.vi"("Task Name"="Test Complete", "Q In"=w340) -> ()  [unwired: 8 in, 2 out]
            n166 = call <vilib>:"Event Log.Record Event.vi"("Message"=w327) -> ()  [unwired: 10 in, 1 out]
            n167 = local write "Status"(w327) -> ()
            n168 = property on="Status" class="Str"("Text.BGColor"=u32 16711680) -> ()  [unwired: 2 in, 2 out]
            n169 = Bundle By Name(cluster=w333, "Test.Running"=FALSE) -> (w332:T13)
          }
          frame "Test Error" {
            n170 = Variant To Data(type="", Variant=w347) -> (data=w344:string, error out=w342:errorcluster)  [unwired: 1 in]
            n171 = call <vilib>:"Scheduler.Clear-Reset.vi"("Q In"=w352) -> ("error out"=w354:errorcluster, "Q Out"=w355:refnum<queue>)  [unwired: 9 in]
            n172 = Flush Queue(queue=w355, error in (no error)=w354) -> (queue out=w356:refnum<queue>)  [unwired: 2 out]
            n173 = Concatenate Strings("Test ERROR!!\n", w344) -> (w343:string)
            n174 = call <vilib>:"Q.Enqueue Task.vi"("Task Name"="Test Complete", "Q In"=w356) -> ()  [unwired: 8 in, 2 out]
            n175 = call <vilib>:"Event Log.Record Event.vi"("Message"=w343) -> ()  [unwired: 10 in, 1 out]
            n176 = local write "Status"(w343) -> ()
            n177 = property on="Status" class="Str"("Text.BGColor"=u32 16711680) -> ()  [unwired: 2 in, 2 out]
            n178 = Bundle By Name(cluster=w349, "Test.Running"=FALSE) -> (w348:T13)
          }
          frame "Test Pass" {
            w358 = "Test PASS"
            n179 = call <vilib>:"Scheduler.Clear-Reset.vi"("Q In"=w363) -> ("error out"=w365:errorcluster, "Q Out"=w366:refnum<queue>)  [unwired: 9 in]
            n180 = Flush Queue(queue=w366, error in (no error)=w365) -> (queue out=w367:refnum<queue>)  [unwired: 2 out]
            n181 = call <vilib>:"Q.Enqueue Task.vi"("Task Name"="Test Complete", "Q In"=w367) -> ()  [unwired: 8 in, 2 out]
            n182 = call <vilib>:"Event Log.Record Event.vi"("Message"=w358) -> ()  [unwired: 10 in, 1 out]
            n183 = local write "Status"(w358) -> ()
            n184 = property on="Status" class="Str"("Text.BGColor"=u32 6618880) -> ()  [unwired: 2 in, 2 out]
            n185 = Bundle By Name(cluster=w360, "Test.Running"=FALSE) -> (w359:T13)
          }
          frame "Test Complete" {
            w388 = FALSE ("Blinking")
            # "Stop Scheduled Items"
            n186 = To Variant(anything=FALSE) -> (Variant=w371:variant)
            n187 = call <vilib>:"Scheduler.Clear-Reset.vi"("Q In"=w389) -> ("error out"=w385:errorcluster, "Q Out"=w384:refnum<queue>)  [unwired: 9 in]
            n188 = call <vilib>:"Q.Enqueue Task.vi"("Data1"=w371, "Task Name"="Run", "Q In"=w370) -> ()  [unwired: 7 in, 2 out]
            n189 = Flush Queue(queue=w384, error in (no error)=w385) -> (queue out=w380:refnum<queue>)  [unwired: 2 out]
            n190 = Current VI's Menubar() -> (w377:refnum<k9>)
            n191 = To Variant(anything=FALSE) -> (Variant=w382:variant)
            n192 = call <vilib>:"Menu.Enable Item.vi"("Enable"=TRUE, "Tag"="Config", "Menu Ref"=w377) -> ()  [unwired: 7 in, 2 out]
            n193 = call <vilib>:"Q.Enqueue Task.vi"("Data1"=w382, "Task Name"="Lock Test Controls", "Q In"=w380) -> ()  [unwired: 7 in, 2 out]
            n194 = call <vilib>:"Event Log.Record Event.vi"("Message"="Test Ended") -> ()  [unwired: 10 in, 1 out]
            n195 = call <vilib>:"High Resolution Relative Seconds.vi"() -> ("relative seconds"=w374:dbl)
            n196 = property on="Test Running" class="Bool (strict)"("Blinking"=w388) -> ()  [unwired: 2 in, 2 out]
            n197 = local write "Test Running"(w388) -> ()
            n198 = Format Date/Time String() -> (date/time string=→"End Time":string)  [unwired: 3 in]
            n199 = local write "Test Ctrl Tab"(enum32{"Idle", "Running", "Completed"}."Completed" ("Test Ctrl Tab")) -> ()
            n200 = Bundle By Name(cluster=w378, "Test.Running"=FALSE ("Running"), "Test.End"=w374) -> (w387:T13)
          }
          frame "Test Reset" {
            # "Clear Data"
            n201 = call <vilib>:"Q.Enqueue Reset.vi"("Q In"=w393) -> ()  [unwired: 9 in, 2 out]
            n202 = invoke on="Results" class="Tbl (strict)" method="Reinit To Default"() -> ()  [unwired: 3 in, 3 out]
            n203 = local write "Status"("Ready") -> ()
            n204 = call <vilib>:"Event Log.Record Event.vi"("Message"="Test Reset") -> ()  [unwired: 10 in, 1 out]
            n205 = property on="Status" class="Str"("Text.BGColor"=u32 13816530) -> ()  [unwired: 2 in, 2 out]
            n206 = invoke on="Start Time" class="Str" method="Reinit To Default"() -> ()  [unwired: 3 in, 3 out]
            n207 = invoke on="End Time" class="Str" method="Reinit To Default"() -> ()  [unwired: 3 in, 3 out]
            n208 = invoke on="UUT PN" class="Str" method="Reinit To Default"() -> ()  [unwired: 3 in, 3 out]
            n209 = invoke on="Rev" class="Str" method="Reinit To Default"() -> ()  [unwired: 3 in, 3 out]
            n210 = invoke on="UUT SN" class="Str" method="Reinit To Default"() -> ()  [unwired: 3 in, 3 out]
            n211 = Bundle By Name(cluster=w396, "Test"=T9 {"Running"=FALSE, "Results"=[], "Start"=0.0, "End"=0.0, "Duration"=0.0, "Failing"=FALSE, "Abort"=FALSE, "TC Level"=0, "TC Cnts"=[], "Test ID"=""}) -> (w395:T13)
            "Test Ctrl Tab" <- enum32{"Idle", "Running", "Completed"}."Idle" ("Test Ctrl Tab")
          }
          frame "TCP-IP Rcv" {
            n212 = Variant To Data(type="", Variant=w410) -> (data=w401:string)  [unwired: 1 in, 1 out]
            n213 = call "TestExec.Script Raw Message to Cluster.vi"("Message Str"=w401) -> ("error out"=w404:errorcluster, "Msg"=w405:T10)  [unwired: 1 in]
            n214 = Unbundle By Name(w405) -> ("Address"=w406:string)
            n215 = case shown="No Error" w404 {
              selector: w404 -> [_ w442]
              tunnel: w407 -> [w415 _]
              tunnel: w402 -> [w418 w444]
              tunnel: w406 -> [w416 _]
              tunnel: w405 -> [w419 w443]
              tunnel: [w413 w441] -> w403
              frame No Error {
                n216 = case shown="Default" w416 {
                  tunnel: w418 -> [w436 w438 w439]
                  tunnel: [w436 w438 w440] -> w417
                  tunnel: w415 -> [_ _ w440]
                  tunnel: [TRUE _ _] -> w414
                  tunnel: [w436 w438 w439] -> w412
                  frame Default {
                    # "Unrecognized"
                  }
                  frame "", "TestExec" {
                  }
                  frame "StationX" {
                  }
                }
                n217 = case shown="False" w414 {
                  tunnel: w419 -> [w430 w432]
                  tunnel: w417 -> [w421 w433]
                  tunnel: [_ w431] -> w413
                  tunnel: w412 -> [w420 _]
                  frame False {
                    w427 = T14 {"Ret Q"=refnum, "Ret Msg"={"Cmd"="", "Sub"="", "Data1"=variant, "Data2"=variant}, "SeqNum"=0}  # Ret Req
                    # "Forward Message"
                    n218 = Unbundle By Name(w430) -> ("Seq"=w423:i32)
                    n219 = Bundle By Name(cluster=w427, "Ret Q"=w420, "Ret Msg.Cmd"="Task", "Ret Msg.Sub"="Data Ret", "SeqNum"=w423) -> (w424:T14)
                    n220 = Unbundle By Name(w430) -> ("Function"=w429:string, "Data"=w428:variant)
                    n221 = call <vilib>:"Q.Enqueue Item.vi"("Data2"=w424, "Data1"=w428, "Sub"=w429, "Cmd"="Function", "Q In"=w421) -> ()  [unwired: 5 in, 2 out]
                  }
                  frame True {
                    # "NAK"
                    n222 = call "TestExec.Script Build Return Message.vi"("Msg"=w432) -> ("error out"=w431:errorcluster, "RetStr"=w435:string)  [unwired: 3 in]
                    n223 = call <vilib>:"Q.Enqueue Task.vi"("Data1"=w435, "Task Name"="TCP-IP Snd", "Q In"=w433) -> ()  [unwired: 7 in, 2 out]
                  }
                }
              }
              frame Error {
                # "NAK"
                n224 = call "TestExec.Script Build Return Message.vi"("error in"=w442, "Msg"=w443) -> ("error out"=w441:errorcluster, "RetStr"=w446:string)  [unwired: 2 in]
                n225 = call <vilib>:"Q.Enqueue Task.vi"("Data1"=w446, "Task Name"="TCP-IP Snd", "Q In"=w444) -> ()  [unwired: 7 in, 2 out]
              }
            }
          }
          frame "TCP-IP Snd" {
            n226 = Variant To Data(type="", Variant=w450) -> (data=w448:string)  [unwired: 1 in, 1 out]
            n227 = call "TCP-IP Mgr.Send.vi"("Send Data"=w448) -> ("error out"=w447:errorcluster)  [unwired: 10 in]
          }
          frame "TCP-IP Connect Event" {
            # "Connect"
            n228 = Variant To Data(type=FALSE, Variant=w458) -> (data=w454:bool)  [unwired: 1 in, 1 out]
            n229 = Unbundle By Name(w456) -> ("Test.Running"=w455:bool)
            n230 = case shown="True" w455 {
              tunnel: w454 -> [w461 w465]
              tunnel: w453 -> [w460 w464]
              frame False {
                n231 = case shown="False" w461 {
                  tunnel: w460 -> [_ w462]
                  frame False {
                  }
                  frame True {
                    n232 = call <vilib>:"Q.Enqueue Task.vi"("Task Name"="Test Reset", "Q In"=w462) -> ()  [unwired: 8 in, 2 out]
                  }
                }
              }
              frame True {
                n233 = case shown="True" w465 {
                  tunnel: w464 -> [w466 _]
                  frame False {
                    n234 = call <vilib>:"Q.Enqueue Task.vi"("Data1"="ERROR!! Connection to Test Sequence was Lost" ("Message"), "Task Name"="Test Abort", "Q In"=w466) -> ()  [unwired: 7 in, 2 out]
                  }
                  frame True {
                    # "Do not allow auto commands to \ninterfere with test in progress.\nDisconnect"
                  }
                }
              }
            }
          }
          frame "Data Ret" {
            n235 = Variant To Data(type=T11 {"SeqNum"=0, "Data"=variant, "Error"={"status"=FALSE, "code"=0, "source"=""}} ("Ret"), Variant=w477) -> (data=w475:T11)  [unwired: 1 in, 1 out]
            n236 = Unbundle By Name(w475) -> ("SeqNum"=w473:i32, "Error"=w472:errorcluster)
            n237 = Bundle By Name(cluster=T10 {"Seq"=0, "Address"="", "Function"="", "Data"=variant, "Error"={"status"=FALSE, "code"=0, "source"=""}} ("Msg"), "Seq"=w473, "Error"=w472) -> (w471:T10)
            n238 = call "TestExec.Script Build Return Message.vi"("Msg"=w471, "Data1"=w476) -> ("error out"=w469:errorcluster, "RetStr"=w470:string)  [unwired: 2 in]
            n239 = call <vilib>:"Q.Enqueue Task.vi"("Data1"=w470, "Task Name"="TCP-IP Snd", "Q In"=w479) -> ()  [unwired: 7 in, 2 out]
          }
          frame "Error Update" {
            w486 = T16 {"Cnt"=0, "Recent Error"={"status"=FALSE, "code"=0, "source"=""}}  # Error Report
            n240 = Variant To Data(type=w486, Variant=w487) -> (data=w485:T16)  [unwired: 1 in, 1 out]
            n241 = Unbundle By Name(w485) -> ("Cnt"=w484:i32)  [unwired: 1 out]
            n242 = Greater Than 0?(x=w484) -> (x > 0?=→"Error":bool)
          }
          frame "Resize" {
            n243 = Unbundle By Name(w492) -> ("Main Tab"=w491:refnum<vi>)
            n244 = control-ref of="Title"() -> (w490:refnum<vi>)
            n245 = while {
              tunnel: w491 -> [w495]
              tunnel: w490 -> [w494]
              i -> [w497]
              stop <- w496 stop-if-true
              n246 = case shown="0" w497 {
                tunnel: [_ TRUE] -> w496
                tunnel: w495 -> [w506 w512]
                tunnel: w494 -> [w498 w511]
                tunnel: [_ w509] -> _
                frame 0 {
                  n247 = property class="TabCtl"(reference=w506) -> ("Width"=w503:u32)  [unwired: 1 in, 2 out]
                  n248 = property class="Str"(reference=w498) -> ("Width"=w502:u32)  [unwired: 1 in, 2 out]
                  n249 = Subtract(x=w503, y=w502) -> (x-y=w501:u32)
                  n250 = Divide(x=w501, y=2) -> (x/y=w500:dbl)
                  n251 = To Long Integer(number=w500) -> (32bit integer=w499:i32)
                  n252 = call <vilib>:"Resize.Align Ctrl within Tab Ctrl.vi"("Child Ref Pos"=T12."Top Left", "dY"=10 ("dX"), "Parent Ref Pos"=T12."Top Left", "dX"=w499, "Child Ctrl"=w498, "Parent Tab Ctrl"=w506) -> ()  [unwired: 3 in, 3 out]
                }
                frame Default {
                  # "Done"
                  n253 = Build Array(w512, w511) -> (w510:refnum<vi>[])
                  n254 = Close Reference(reference=w510) -> (error out=w509:errorcluster)  [unwired: 1 in]
                }
              }
            }
          }
          frame Default {
            n255 = call <vilib>:"Module.Default Tasks.vi"("Sys"=w519, "error in"=w515, "Data2"=w516, "Data1"=w517, "Sub"=w518) -> ("error out"=w514:errorcluster)  [unwired: 6 in]
          }
        }
      }
      frame "Function" {
        n256 = case shown="\"TestSection_Start\"" w528 {
          selector: w528 -> [_ _ _ _ _ _ _ w647 _]
          tunnel: w532 -> [w541 w560 w584 w594 w618 w628 w640 w651 w659]
          tunnel: w531 -> [w535 w555 w576 w588 w612 w627 w639 w652 w657]
          tunnel: [w541 w560 w584 w594 w618 w628 w640 w651 w659] -> w530
          tunnel: [w534 w554 w577 w587 w611 w627 w639 w652 w657] -> w529
          tunnel: w527 -> [w540 w559 _ w593 _ w626 w638 _ _]
          tunnel: w526 -> [w533 _ _ _ _ w624 w635 _ w658]
          tunnel: w525 -> [_ _ _ _ _ _ _ _ _]
          tunnel: w523 -> [_ _ _ _ _ _ _ _ _]
          tunnel: [w537 w556 _ w590 _ w621 w632 w644 _] -> w522
          tunnel: [_ w552 w574 w586 w610 _ _ variant _] -> w521
          frame "TestStart" {
            # "Test Name, Version"
            n257 = Variant To Data(type=string[] [], Variant=w540) -> (data=w536:string[], error out=w538:errorcluster)  [unwired: 1 in]
            n258 = case shown="No Error" w538 {
              selector: w538 -> [_ w550]
              tunnel: [_ w549] -> w537
              tunnel: w536 -> [w545 _]
              tunnel: w535 -> [w542 w547]
              tunnel: [w542 w547] -> w534
              tunnel: w533 -> [w546 _]
              frame No Error {
                n259 = To Variant(anything=w545) -> (Variant=w544:variant)
                n260 = call <vilib>:"Q.Enqueue Task.vi"("Data1"=w544, "Task Name"="Test Start", "Q In"=w546) -> ()  [unwired: 7 in, 2 out]
              }
              frame Error {
                n261 = Bundle By Name(cluster=w550, "source"="Invalid parameter data type.  Expected Array of String.") -> (w549:errorcluster)
              }
            }
          }
          frame "TestSection_Start" {
            n262 = Variant To Data(type="", Variant=w559) -> (data=w553:string, error out=w557:errorcluster)  [unwired: 1 in]
            n263 = case shown="No Error" w557 {
              selector: w557 -> [_ w573]
              tunnel: [_ w572] -> w556
              tunnel: w555 -> [w564 w570]
              tunnel: [w563 w570] -> w554
              tunnel: w553 -> [w562 _]
              tunnel: [w561 _] -> w551
              frame No Error {
                n264 = Unbundle By Name(w564) -> ("ResultID"=w566:refnum<class "Class - ResultCntr.lvclass">)
                n265 = call "Class - ResultCntr.SectionStart.vi"("Class - ResultCntr in"=w566) -> ("ID"=w561:string, "Class - ResultCntr out"=w565:refnum<class "Class - ResultCntr.lvclass">)  [unwired: 8 in, 1 out]
                n266 = local read "Results"() -> (w569:string[][])
                n267 = Build Array(w561, w562) -> (w568:string[])
                n268 = Bundle By Name(cluster=w564, "ResultID"=w565) -> (w563:T13)
                n269 = Build Array (concatenate)(w569, w568) -> (→"Results":string[][])
              }
              frame Error {
                n270 = Bundle By Name(cluster=w573, "source"="Invalid parameter data type.  Expected string.") -> (w572:errorcluster)
              }
            }
            n271 = To Variant(anything=w551) -> (Variant=w552:variant)
          }
          frame "TestSection_End" {
            n272 = Unbundle By Name(w576) -> ("ResultID"=w579:refnum<class "Class - ResultCntr.lvclass">)
            n273 = call "Class - ResultCntr.SectionEnd.vi"("Class - ResultCntr in"=w579) -> ("ID"=w575:string, "Class - ResultCntr out"=w578:refnum<class "Class - ResultCntr.lvclass">)  [unwired: 8 in, 1 out]
            n274 = local read "Results"() -> (w583:string[][])
            n275 = Build Array(w575, "Section End" ("Task Name")) -> (w582:string[])
            n276 = Bundle By Name(cluster=w576, "ResultID"=w578, "Test.Test ID"=w575) -> (w577:T13)
            n277 = Build Array (concatenate)(w583, w582) -> (w581:string[][])
            n278 = local write "Results"(w581) -> ()
            n279 = To Variant(anything=w575) -> (Variant=w574:variant)
          }
          frame "TestSubsection_Start" {
            n280 = Variant To Data(type="", Variant=w593) -> (data=w589:string, error out=w591:errorcluster)  [unwired: 1 in]
            n281 = case shown="No Error" w591 {
              selector: w591 -> [_ w607]
              tunnel: [_ w606] -> w590
              tunnel: w589 -> [w595 _]
              tunnel: w588 -> [w598 w604]
              tunnel: [w597 w604] -> w587
              tunnel: [w596 _] -> w585
              frame No Error {
                n282 = Unbundle By Name(w598) -> ("ResultID"=w601:refnum<class "Class - ResultCntr.lvclass">)
                n283 = call "Class - ResultCntr.SubSectionStart.vi"("Class - ResultCntr in"=w601) -> ("ID"=w596:string, "Class - ResultCntr out"=w600:refnum<class "Class - ResultCntr.lvclass">)  [unwired: 8 in, 1 out]
                n284 = local read "Results"() -> (w603:string[][])
                n285 = Build Array(w596, w595) -> (w602:string[])
                n286 = Bundle By Name(cluster=w598, "ResultID"=w600) -> (w597:T13)
                n287 = Build Array (concatenate)(w603, w602) -> (w599:string[][])
                n288 = local write "Results"(w599) -> ()
              }
              frame Error {
                n289 = Bundle By Name(cluster=w607, "source"="Invalid parameter data type.  Expected string.") -> (w606:errorcluster)
              }
            }
            n290 = To Variant(anything=w585) -> (Variant=w586:variant)
          }
          frame "TestSubsection_End" {
            n291 = Unbundle By Name(w612) -> ("ResultID"=w615:refnum<class "Class - ResultCntr.lvclass">)
            n292 = call "Class - ResultCntr.SubSectionEnd.vi"("Class - ResultCntr in"=w615) -> ("ID"=w609:string, "Class - ResultCntr out"=w614:refnum<class "Class - ResultCntr.lvclass">)  [unwired: 8 in, 1 out]
            n293 = local read "Results"() -> (w617:string[][])
            n294 = Build Array(w609, "Section End") -> (w616:string[])
            n295 = Bundle By Name(cluster=w612, "ResultID"=w614) -> (w611:T13)
            n296 = Build Array (concatenate)(w617, w616) -> (w613:string[][])
            n297 = local write "Results"(w613) -> ()
            n298 = To Variant(anything=w609) -> (Variant=w610:variant)
          }
          frame "TestResultFloat" {
            n299 = Variant To Data(type=string[] [], Variant=w626) -> (data=w620:string[], error out=w622:errorcluster)  [unwired: 1 in]
            n300 = To Variant(anything=w620) -> (Variant=w619:variant)
            n301 = call <vilib>:"Q.Enqueue Task.vi"("Data1"=w619, "Task Name"="TestResultFloat", "Q In"=w624) -> ()  [unwired: 7 in, 2 out]
            n302 = case shown="No Error" w622 {
              selector: w622 -> [_ w631]
              tunnel: [_ w630] -> w621
              frame No Error {
              }
              frame Error {
                n303 = Bundle By Name(cluster=w631, "source"="Invalid parameter data type.  Expected Array of String.") -> (w630:errorcluster)
              }
            }
          }
          frame "TestError" {
            # "Section Name"
            n304 = Variant To Data(type="", Variant=w638) -> (data=w634:string, error out=w633:errorcluster)  [unwired: 1 in]
            n305 = call <vilib>:"Q.Enqueue Task.vi"("Data1"=w634, "Task Name"="Test Error", "Q In"=w635) -> ()  [unwired: 7 in, 2 out]
            n306 = case shown="Error" w633 {
              selector: w633 -> [_ w643]
              tunnel: [_ w642] -> w632
              frame No Error {
              }
              frame Error {
                n307 = Bundle By Name(cluster=w643, "source"="Invalid parameter data type.  Expected string.") -> (w642:errorcluster)
              }
            }
          }
          frame Default {
            n308 = Concatenate Strings("Unrecognized function: \"" ("source"), w647, "\"." ("source")) -> (w645:string)
            n309 = Bundle By Name(cluster=errorcluster {"status"=TRUE, "code"=-5000, "source"=" "} ("error constant"), "source"=w645) -> (w644:errorcluster)
          }
          frame "TestComplete" {
            n310 = Unbundle By Name(w657) -> ("Test.Failing"=w656:bool)
            n311 = Select(t="Test Fail" ("Task Name"), s=w656, f="Test Pass" ("Task Name")) -> (s? t:f=w653:string)
            n312 = call <vilib>:"Q.Enqueue Task.vi"("Task Name"=w653, "Q In"=w658) -> ()  [unwired: 8 in, 2 out]
          }
        }
        n313 = call <vilib>:"Q.Return Function Data.vi"("error in"=w522, "Data2"=w523, "Ret Data"=w521) -> ("error out"=w524:errorcluster)  [unwired: 8 in]
      }
      frame "Error", Default {
        n314 = Unbundle By Name(w662) -> ("Test.Running"=w663:bool)
        n315 = case shown="\"Error\"" w668 {
          selector: w668 -> [_ w705]
          tunnel: [w673 w706] -> w669
          tunnel: w667 -> [w678 _]
          tunnel: w666 -> [w676 _]
          tunnel: w665 -> [w677 _]
          tunnel: w664 -> [w675 _]
          tunnel: w663 -> [w671 _]
          frame "Error" {
            n316 = case shown="\"Error\"" w677 {
              tunnel: w678 -> [_ w704]
              tunnel: w676 -> [w700 _]
              tunnel: [w700 w702] -> w672
              tunnel: w675 -> [w699 w701]
              tunnel: [w699 w701] -> w674
              frame Default {
              }
              frame "Error" {
                n317 = Variant To Data(type=errorcluster {"status"=FALSE, "code"=0, "source"=""} ("error constant"), Variant=w704) -> (data=w702:errorcluster)  [unwired: 1 in, 1 out]
              }
            }
            n318 = case shown="False" w671 {
              tunnel: w674 -> [w682 w697]
              tunnel: [w681 w690] -> w673
              tunnel: w672 -> [w679 w696]
              frame False {
                n319 = call <vilib>:"Event Log.Record Event.vi"("error in"=w679) -> ()  [unwired: 10 in, 1 out]
                n320 = case shown="\"Ignore\"" enum16{"Exit", "Reset", "Ignore"}."Ignore" ("Selection") {
                  tunnel: w682 -> [w684 _ w689]
                  tunnel: [w683 _ w688] -> w681
                  tunnel: w679 -> [_ w687 _]
                  frame "Exit", Default {
                    n321 = call <vilib>:"Q.Enqueue Exit.vi"("Q In"=w684) -> ("error out"=w683:errorcluster)  [unwired: 9 in, 1 out]
                  }
                  frame "Ignore" {
                    w685 = TRUE ("Error")
                    n322 = Unbundle By Name(w687) -> ("source"=w686:string)
                    n323 = property on="Error" class="Bool (strict)"("Visible"=w685, "TipStrip"=w686) -> ()  [unwired: 2 in, 2 out]
                    "Error" <- w685
                  }
                  frame "Reset" {
                    n324 = call <vilib>:"Q.Enqueue Reset.vi"("Q In"=w689) -> ("error out"=w688:errorcluster)  [unwired: 9 in, 1 out]
                  }
                }
              }
              frame True {
                n325 = Unbundle By Name(w696) -> ("code"=w693:i32, "source"=w692:string)
                n326 = Format Into String(format string="\nCode: %d\nDescription: %s" ("Message"), initial string="Test Aborted due to ERROR!!" ("Message"), w693, w692) -> (resulting string=w691:string, error out=w690:errorcluster)  [unwired: 1 in]
                n327 = call <vilib>:"Q.Enqueue Task.vi"("Data1"=w691, "Task Name"="Test Abort", "Q In"=w697) -> ()  [unwired: 7 in, 2 out]
              }
            }
          }
          frame Default {
            n328 = Concatenate Strings("Undefined State: \"", w705, "\".") -> (w707:string)
            n329 = Bundle By Name(cluster=errorcluster {"status"=TRUE, "code"=-5000, "source"=""} ("error constant"), "source"=w707) -> (w706:errorcluster)
          }
        }
        n330 = Bundle By Name(cluster=w662, "Test.Running"=FALSE) -> (w661:T13)
      }
      frame "Exit" {
        # "Save control states"
        n331 = Unbundle By Name(w715) -> ("CtrlStates"=w713:refnum<class "Class.SaveCtrls.lvclass">)
        n332 = call <vilib>:"Q.Enqueue Exit.vi"("Q In"=w712) -> ()  [unwired: 9 in, 2 out]
        n333 = call "TCP-IP Mgr.Destroy.vi"() -> ("error out"=w711:errorcluster)  [unwired: 11 in]
        n334 = call-dynamic "Class.SaveCtrls.Save.vi"("CtrlStates In"=w713) -> ("error out"=w714:errorcluster)  [unwired: 9 in, 1 out]
        n335 = call <vilib>:"Clear Errors.vi"("error in (no error)"=w714) -> ()  [unwired: 5 in, 2 out]
        n336 = call <vilib>:"Clear Errors.vi"("error in (no error)"=w711) -> ()  [unwired: 5 in, 2 out]
        n337 = call <vilib>:"Module.Destructor.vi"("Sys"=w716) -> ("error out"=w718:errorcluster)  [unwired: 10 in]
      }
    }
  }
  n338 = while {
    tunnel: w5 -> [w731]
    shift-right: [w726] -> _
    shift-left: w8 -> [w730]
    tunnel: w4 -> [w725]
    shift-right: [w723] -> _
    shift-left: _ -> [w724]
    stop <- w722 stop-if-true
    n339 = call <vilib>:"Q.Dequeue + Error Check.vi"("Error In"=w730, "Q In"=w731) -> ("error out"=w727:errorcluster, "Cmd"=w729:string, "Q Out"=w728:refnum<queue>, "Data1"=w720:variant, "Sub"=w721:string, "Data2"=w719:variant)  [unwired: 4 in]
    n340 = case shown="\"Task\"" w729 {
      tunnel: w728 -> [_ w739 _ w766 w845 _]
      tunnel: w727 -> [w733 w738 _ _ _ _]
      tunnel: [w737 _ _ w765 w844 _] -> w726
      tunnel: w725 -> [w735 _ _ _ _ _]
      tunnel: w724 -> [w736 _ w759 w771 w849 w913]
      tunnel: [w736 w741 w760 w770 w848 w913] -> w723
      tunnel: [_ _ _ _ _ TRUE] -> w722
      tunnel: w721 -> [_ _ _ w769 w847 _]
      tunnel: w720 -> [_ _ _ w768 w846 _]
      tunnel: w719 -> [_ _ _ w767 w842 _]
      frame "Error", Default {
        n341 = To Variant(anything=w733) -> (Variant=w732:variant)
        n342 = call <vilib>:"Q.Enqueue Item.vi"("Data1"=w732, "Cmd"="Error", "Q In"=w735) -> ("error out"=w737:errorcluster)  [unwired: 7 in, 1 out]
      }
      frame "Init" {
        w742 = FALSE  # Running
        n343 = call <vilib>:"Q.Enqueue Reset.vi"("Top of Q(T)"=TRUE ("Flush Q"), "Error In"=w738, "Q In"=w739) -> ()  [unwired: 7 in, 2 out]
        n344 = Bundle("Running"=w742) -> (w741:cluster{"Running":bool})  [unwired: 1 in]
      }
      frame "Reset" {
        w743 = FALSE ("Running")
        n345 = for {
          N: 4 -> [_]
          tunnel: [w764] -> w749 mode=indexing
          n346 = Random Number (0-1)() -> (number: 0 to 1=w764:dbl)
        }
        n347 = invoke on="Output Hist" class="WFChart (strict)" method="Reinit To Default"() -> ()  [unwired: 3 in, 3 out]
        n348 = invoke on="UUT State" class="Clust (strict)" method="Reinit To Default"() -> ()  [unwired: 3 in, 3 out]
        n349 = invoke on="OutputX" class="DigNum (strict)" method="Reinit To Default"() -> ()  [unwired: 3 in, 3 out]
        n350 = invoke on="OutputY" class="DigNum (strict)" method="Reinit To Default"() -> ()  [unwired: 3 in, 3 out]
        n351 = Greater Or Equal?(x=w749, y=0.5) -> (x >= y?=→"Data1DBool":bool[])
        n352 = for {
          N: 2 -> [_]
          tunnel: [w761] -> w745 mode=indexing
          n353 = for {
            N: 2 -> [_]
            tunnel: [w763] -> w761 mode=indexing
            n354 = Random Number (0-1)() -> (number: 0 to 1=w763:dbl)
          }
        }
        n355 = Initialize Array(3.0 ("element"), 4 ("dimension size")) -> (→"Data1DFloat":dbl[])
        n356 = Initialize Array(6.0 ("element"), 2 ("dimension size"), 4 ("dimension size")) -> (→"Data2DFloat":dbl[][])
        n357 = Greater Or Equal?(x=w745, y=0.5) -> (x >= y?=→"Data2DBool":bool[][])
        n358 = Bundle By Name(cluster=w759, "Running"=w743) -> (w760:cluster{"Running":bool})
        n359 = local write "ON/OFF"(w743) -> ()
      }
      frame "Task" {
        n360 = case shown="\"UUTPower\"" w769 {
          selector: w769 -> [_ w775 _ _ _]
          tunnel: w771 -> [w772 w774 w814 w827 w830]
          tunnel: [w772 w774 w813 w827 w830] -> w770
          tunnel: w768 -> [_ _ w812 _ w834]
          tunnel: w767 -> [_ _ _ _ _]
          tunnel: w766 -> [_ w776 w810 _ _]
          tunnel: [_ _ w807 _ w831] -> w765
          frame Default {
          }
          frame "Update" {
            n361 = Unbundle By Name(w774) -> ("Running"=w773:bool)
            n362 = case shown="True" w773 {
              tunnel: w776 -> [_ w794]
              tunnel: w775 -> [_ w793]
              frame False {
              }
              frame True {
                n363 = call <vilib>:"Scheduler.AddTask.vi"("Interval(s)"=0.2, "Task Name"=w793, "Sched Name"=w793, "Q In"=w794) -> ()  [unwired: 6 in, 2 out]
              }
            }
            n364 = local read "Data2DFloat"() -> (w777:dbl[][])
            n365 = local read "Data1DFloat"() -> (w779:dbl[])
            n366 = for {
              tunnel: w777 -> [w796] mode=indexing
              tunnel: [w795] -> w778 mode=indexing
              n367 = for {
                tunnel: w796 -> [w801] mode=indexing
                tunnel: [w797] -> w795 mode=indexing
                n368 = Random Number (0-1)() -> (number: 0 to 1=w800:dbl)
                n369 = Subtract(x=w800, y=0.5) -> (x-y=w798:dbl)
                n370 = Add(x=w801, y=w798) -> (x+y=w797:dbl)
              }
            }
            n371 = for {
              tunnel: w779 -> [w806] mode=indexing
              tunnel: [w802] -> w780 mode=indexing
              n372 = Random Number (0-1)() -> (number: 0 to 1=w805:dbl)
              n373 = Subtract(x=w805, y=0.5) -> (x-y=w803:dbl)
              n374 = Add(x=w806, y=w803) -> (x+y=w802:dbl)
            }
            n375 = local write "Data1DFloat"(w780) -> ()
            n376 = local write "Data2DFloat"(w778) -> ()
            n377 = Random Number (0-1)() -> (number: 0 to 1=w786:dbl)
            n378 = Random Number (0-1)() -> (number: 0 to 1=w783:dbl)
            n379 = Multiply(x=0.5, y=w786) -> (x*y=w787:dbl)
            n380 = Multiply(x=0.5, y=w783) -> (x*y=w782:dbl)
            n381 = Add(x=w787, y=3.3) -> (x+y=w791:dbl)
            "OutputY" <- w791
            n382 = Add(x=w782, y=5.0) -> (x+y=w790:dbl)
            "OutputX" <- w790
            n383 = Bundle(w790, w791) -> (→"Output Hist":cluster{dbl, dbl})  [unwired: 1 in]
          }
          frame "UUTPower" {
            n384 = Variant To Data(type=FALSE, Variant=w812) -> (data=w808:bool, error out=w807:errorcluster)  [unwired: 1 in]
            n385 = case shown="True" w808 {
              tunnel: w810 -> [w818 w823]
              tunnel: [T2 {"Standby"=TRUE, "Initializing"=FALSE, "Running"=FALSE, "Error"=FALSE} ("UUT State") T2 {"Standby"=FALSE, "Initializing"=TRUE, "Running"=FALSE, "Error"=FALSE} ("UUT State")] -> w809
              frame False {
                n386 = call <vilib>:"Scheduler.Delete Task.vi"("Sched Name"="Update" ("Task Name"), "Q In"=w818) -> ("Q Out"=w816:refnum<queue>)  [unwired: 8 in, 1 out]
                n387 = call <vilib>:"Scheduler.Delete Task.vi"("Sched Name"="Init Done" ("Task Name"), "Q In"=w816) -> ()  [unwired: 8 in, 2 out]
              }
              frame True {
                w822 = "Update" ("Task Name")
                w825 = "Init Done" ("Task Name")
                n388 = call <vilib>:"Scheduler.AddTask.vi"("Interval(s)"=2.0, "Task Name"=w822, "Sched Name"=w822, "Q In"=w823) -> ("Q Out"=w824:refnum<queue>)  [unwired: 6 in, 1 out]
                n389 = call <vilib>:"Scheduler.AddTask.vi"("Interval(s)"=2.0, "Task Name"=w825, "Sched Name"=w825, "Q In"=w824) -> ()  [unwired: 6 in, 2 out]
              }
            }
            "UUT State" <- w809
            n390 = Bundle By Name(cluster=w814, "Running"=w808) -> (w813:cluster{"Running":bool})
          }
          frame "Init Done" {
            n391 = local write "UUT State"(T2 {"Standby"=FALSE, "Initializing"=FALSE, "Running"=TRUE, "Error"=FALSE} ("UUT State")) -> ()
          }
          frame "UUT Error" {
            n392 = Variant To Data(type=FALSE, Variant=w834) -> (data=w832:bool, error out=w831:errorcluster)  [unwired: 1 in]
            n393 = Unbundle By Name(w830) -> ("Running"=w829:bool)
            n394 = case shown="False" w829 {
              tunnel: [T2 {"Standby"=TRUE, "Initializing"=FALSE, "Running"=FALSE, "Error"=FALSE} ("UUT State") w838] -> w835
              tunnel: w832 -> [_ w837]
              frame False {
              }
              frame True {
                n395 = case shown="False" w837 {
                  tunnel: [T2 {"Standby"=FALSE, "Initializing"=FALSE, "Running"=TRUE, "Error"=FALSE} ("UUT State") T2 {"Standby"=FALSE, "Initializing"=FALSE, "Running"=FALSE, "Error"=TRUE} ("UUT State")] -> w838
                  frame False {
                  }
                  frame True {
                  }
                }
              }
            }
            n396 = local write "UUT State"(w835) -> ()
          }
        }
      }
      frame "Function" {
        n397 = case shown="\"SetUUTPower\"" w847 {
          selector: w847 -> [_ _ _ _ _ _ _ _ _ _ w905]
          tunnel: w849 -> [w857 w869 w872 w883 w886 w889 w892 w895 w898 w901 w904]
          tunnel: [w856 w869 w872 w883 w886 w889 w892 w895 w898 w901 w904] -> w848
          tunnel: w846 -> [w855 _ _ _ _ _ _ _ _ _ _]
          tunnel: w842 -> [_ _ _ _ _ _ _ _ _ _ _]
          tunnel: w845 -> [w852 _ _ _ _ _ _ _ _ _ _]
          tunnel: [w853 _ _ _ _ _ _ _ _ _ w906] -> w843
          tunnel: [_ w871 w873 w885 w888 w891 w894 w897 w900 w903 variant] -> w841
          frame "SetUUTPower" {
            n398 = Variant To Data(type=FALSE, Variant=w855) -> (data=w850:bool, error out=w853:errorcluster)  [unwired: 1 in]
            n399 = case shown="True" w850 {
              tunnel: w852 -> [w861 w865]
              tunnel: [T2 {"Standby"=TRUE, "Initializing"=FALSE, "Running"=FALSE, "Error"=FALSE} ("UUT State") T2 {"Standby"=FALSE, "Initializing"=TRUE, "Running"=FALSE, "Error"=FALSE} ("UUT State")] -> w851
              frame False {
                n400 = call <vilib>:"Scheduler.Delete Task.vi"("Sched Name"="Update" ("Task Name"), "Q In"=w861) -> ("Q Out"=w859:refnum<queue>)  [unwired: 8 in, 1 out]
                n401 = call <vilib>:"Scheduler.Delete Task.vi"("Sched Name"="Init Done" ("Task Name"), "Q In"=w859) -> ()  [unwired: 8 in, 2 out]
              }
              frame True {
                w867 = "Init Done" ("Task Name")
                w864 = 2.0 ("Interval(s)")
                w863 = "Update" ("Task Name")
                n402 = call <vilib>:"Scheduler.AddTask.vi"("Interval(s)"=w864, "Task Name"=w863, "Sched Name"=w863, "Q In"=w865) -> ("Q Out"=w866:refnum<queue>)  [unwired: 6 in, 1 out]
                n403 = call <vilib>:"Scheduler.AddTask.vi"("Interval(s)"=w864, "Task Name"=w867, "Sched Name"=w867, "Q In"=w866) -> ()  [unwired: 6 in, 2 out]
              }
            }
            n404 = local write "ON/OFF"(w850) -> ()
            n405 = local write "UUT State"(w851) -> ()
            n406 = Bundle By Name(cluster=w857, "Running"=w850) -> (w856:cluster{"Running":bool})
          }
          frame "GetONOFF" {
            n407 = local read "ON/OFF"() -> (w870:bool)
            n408 = To Variant(anything=w870) -> (Variant=w871:variant)
          }
          frame "GetUUTState" {
            n409 = local read "UUT State"() -> (w874:T2)
            n410 = Unbundle By Name(w874) -> ("Standby"=w875:bool, "Initializing"=w876:bool, "Running"=w877:bool, "Error"=w878:bool)
            n411 = Build Array(w875, w876, w877, w878) -> (w879:bool[])
            n412 = for {
              tunnel: w879 -> [w882] mode=indexing
              tunnel: [w881] -> w880
              i -> [w881]
              stop <- w882 stop-if-true
            }
            n413 = To Variant(anything=w880) -> (Variant=w873:variant)
          }
          frame "GetOutputX" {
            n414 = local read "OutputX"() -> (w884:dbl)
            n415 = To Variant(anything=w884) -> (Variant=w885:variant)
          }
          frame "GetOutputY" {
            n416 = local read "OutputY"() -> (w887:dbl)
            n417 = To Variant(anything=w887) -> (Variant=w888:variant)
          }
          frame "Get1DBool" {
            n418 = local read "Data1DBool"() -> (w890:bool[])
            n419 = To Variant(anything=w890) -> (Variant=w891:variant)
          }
          frame "Get2DBool" {
            n420 = local read "Data2DBool"() -> (w893:bool[][])
            n421 = To Variant(anything=w893) -> (Variant=w894:variant)
          }
          frame "Get1DFloat" {
            n422 = local read "Data1DFloat"() -> (w896:dbl[])
            n423 = To Variant(anything=w896) -> (Variant=w897:variant)
          }
          frame "Get2DFloat" {
            n424 = local read "Data2DFloat"() -> (w899:dbl[][])
            n425 = To Variant(anything=w899) -> (Variant=w900:variant)
          }
          frame "Get2DStr" {
            n426 = local read "Data2DStr"() -> (w902:string[][])
            n427 = To Variant(anything=w902) -> (Variant=w903:variant)
          }
          frame Default {
            n428 = Concatenate Strings("Unrecognized function: \"" ("source"), w905, "\"." ("source")) -> (w910:string)
            n429 = Bundle By Name(cluster=errorcluster {"status"=TRUE, "code"=-5000, "source"=" "} ("error constant"), "source"=w910) -> (w906:errorcluster)
          }
        }
        n430 = call <vilib>:"Q.Return Function Data.vi"("error in"=w843, "Data2"=w842, "Ret Data"=w841) -> ("error out"=w844:errorcluster)  [unwired: 8 in]
      }
      frame "Exit" {
      }
    }
  }
  n431 = while "Event Loop" {
    tunnel: w9 -> [w919]
    tunnel: w12 -> [_]
    tunnel: w11 -> [w916]
    tunnel: w10 -> [w915]
    tunnel: w5 -> [w914]
    stop <- w920 stop-if-true
    # "UUT"
    # "Power - Update Config"
    n432 = Unbundle By Name(w919) -> ("Stop.Ref"=w918:refnum<event-registration>, "Main Q"=w917:refnum<queue>)
    n433 = event shown="[1] Panel Resize" {
      selector: w918 -> [_ _ _ _ _ _ _ _ _ _ _]
      dyn-events: _ -> [_ _ _ _ _ _ _ _ _ _ _]
      timeout: _ -> [_ _ _ _ _ _ _ _ _ _ _]
      tunnel: [w923 _ _ _ _ w950 TRUE _ _ _ _] -> w920
      tunnel: w919 -> [w922 _ _ _ _ w948 _ _ _ _ _]
      tunnel: w917 -> [w925 w935 w937 w939 _ w949 _ w981 w983 w986 _]
      tunnel: w916 -> [_ _ _ _ _ w941 _ _ _ _ _]
      tunnel: w915 -> [_ _ _ _ _ w942 _ _ _ _ _]
      tunnel: w914 -> [_ _ _ _ _ _ _ _ _ _ w988]
      event Panel Close? {
        n434 = event-data() -> ()  [unwired: 1 in, 4 out]
        n435 = Unbundle By Name(w922) -> ("Cfg.Is Child?"=w921:bool)
        n436 = case shown="False" w921 {
          tunnel: w925 -> [w928 w931]
          tunnel: [TRUE TRUE] -> w924
          tunnel: [TRUE FALSE] -> w923
          tunnel: [_ w929] -> _
          frame False {
            # "Parent - Exit"
            n437 = call <vilib>:"Q.Enqueue Exit.vi"("Q In"=w928) -> ()  [unwired: 9 in, 2 out]
          }
          frame True {
            # "Child - Hide Panel"
            n438 = call <vilib>:"Module.Window, Q Task.vi"("Action"=Window.Task,_Action."Return to SubPanel()", "Q In"=w931) -> ("error out"=w929:errorcluster)  [unwired: 8 in, 1 out]
          }
        }
        n439 = event-data("Discard?"=w924) -> ()  [unwired: 1 in, 1 out]
      }
      event Panel Resize {
        n440 = event-data() -> ()  [unwired: 1 in, 8 out]
        n441 = call <vilib>:"Module.Window, Q Task.vi"("Action"=Window.Task,_Action."Resize()", "Q In"=w935) -> ()  [unwired: 8 in, 2 out]
      }
      event "Show Block Diagram": Value Change {
        n442 = event-data() -> ()  [unwired: 1 in, 6 out]
        n443 = call <vilib>:"Module.Window, Q Task.vi"("Action"=Window.Task,_Action."Open Block Diagram()", "Q In"=w937) -> ()  [unwired: 8 in, 2 out]
      }
      event "Maint": Value Change {
        n444 = event-data() -> ()  [unwired: 1 in, 6 out]
        n445 = call <vilib>:"Module.Window, Q Task.vi"("Action"=Window.Task,_Action."Go To Maint Tab()", "Q In"=w939) -> ()  [unwired: 8 in, 2 out]
      }
      event "Leave Maint": Value Change {
        n446 = event-data() -> ()  [unwired: 1 in, 6 out]
        n447 = local write "Main Tab"(0) -> ()
      }
      event Menu Selection (User) {
        n448 = event-data() -> ("ItemTag"=w943:string)  [unwired: 1 in, 6 out]
        n449 = Match Pattern(string=w943, regular expression="Manuals_") -> (match substring=w945:string, offset past match=w946:i32)  [unwired: 1 in, 2 out]
        n450 = case shown="0, Default" w946 {
          tunnel: w943 -> [_ w952]
          tunnel: [w951 w952] -> w944
          tunnel: w945 -> [w951 _]
          frame 0, Default {
          }
          frame -1 {
          }
        }
        n451 = case shown="\"Show Station UI\"" w944 {
          tunnel: [_ TRUE _ _ _ _ _ _ _ _] -> w950
          tunnel: w949 -> [_ w953 _ _ _ w958 _ _ _ w970]
          tunnel: [_ _ w955 w956 w957 _ w959 _ w969 _] -> _
          tunnel: w948 -> [_ _ _ _ _ _ w960 w963 _ _]
          tunnel: w943 -> [_ _ _ _ _ _ _ _ w965 _]
          tunnel: w942 -> [_ _ _ _ _ _ _ _ w967 _]
          tunnel: w941 -> [_ _ _ _ _ _ _ _ w966 _]
          frame Default {
          }
          frame "Exit" {
            n452 = call <vilib>:"Q.Enqueue Exit.vi"("Q In"=w953) -> ()  [unwired: 9 in, 2 out]
          }
          frame "Show Event Log" {
            n453 = call <vilib>:"Event Log.Show.vi"() -> ("error out"=w955:errorcluster)  [unwired: 11 in]
          }
          frame "Show TCP-IP Log" {
            n454 = call "TCP-IP Mgr.Show.vi"() -> ("error out"=w956:errorcluster)  [unwired: 11 in]
          }
          frame "Show Station UI" {
            n455 = call "TCP-IP Mgr.Show.vi"() -> ("error out"=w957:errorcluster)  [unwired: 11 in]
          }
          frame "Reset" {
            n456 = call <vilib>:"Q.Enqueue Reset.vi"("Q In"=w958) -> ()  [unwired: 9 in, 2 out]
          }
          frame "Open Log Folder" {
            n457 = Unbundle By Name(w960) -> ("Cfg.Dirs.Logs"=w961:path)
            n458 = call <vilib>:"File.Open File or Folder.vi"("Path"=w961) -> ("Error Out"=w959:errorcluster)  [unwired: 10 in]
          }
          frame "Help.About" {
            n459 = Unbundle By Name(w963) -> ("SW Rev"=w962:T5)
            n460 = call "Help.About.vi"("SW Version"=w962) -> ()  [unwired: 11 in]
          }
          frame "Manuals_" {
            n461 = Search 1D Array(1D array=w966, element=w965) -> (index of element=w968:i32)  [unwired: 1 in]
            n462 = Index Array(array=w967, index=w968) -> (element=w964:path)
            n463 = call <vilib>:"File.Open File or Folder.vi"("Path"=w964) -> ("Error Out"=w969:errorcluster)  [unwired: 10 in]
          }
          frame "Config.PowerMeas" {
            n464 = call <vilib>:"Q.Enqueue Task.vi"("Task Name"="Power - Config Dialog", "Q In"=w970) -> ()  [unwired: 8 in, 2 out]
          }
        }
      }
      event User Event {
        n465 = event-data() -> ()  [unwired: 1 in, 5 out]
      }
      event "Start": Value Change {
        # "TODO - Set Timeout if sequence does not connect"
        n466 = event-data() -> ()  [unwired: 1 in, 6 out]
        n467 = To Variant(anything=TRUE) -> (Variant=w974:variant)
        n468 = call <vilib>:"Q.Enqueue Task.vi"("Data1"=w974, "Task Name"="Lock Test Controls", "Q In"=w981) -> ("Q Out"=w976:refnum<queue>)  [unwired: 7 in, 1 out]
        n469 = call <vilib>:"Q.Enqueue Task.vi"("Task Name"="Launch Test Script", "Q In"=w976) -> ()  [unwired: 8 in, 2 out]
        n470 = property on="Test Running" class="Bool (strict)"("Blinking"=TRUE) -> ()  [unwired: 2 in, 2 out]
        "Progress" <- 0.0 ("Progress")
        "Test Running" <- TRUE ("Test Running")
      }
      event "Abort": Value Change {
        n471 = event-data() -> ()  [unwired: 1 in, 6 out]
        n472 = call <vilib>:"Q.Enqueue Task.vi"("Data1"="Test Aborted by Operator" ("Message"), "Task Name"="Test Abort", "Q In"=w983) -> ()  [unwired: 7 in, 2 out]
      }
      event "Test Reset": Value Change {
        n473 = event-data() -> ()  [unwired: 1 in, 6 out]
        n474 = call <vilib>:"Q.Enqueue Task.vi"("Task Name"="Test Reset", "Q In"=w986) -> ()  [unwired: 8 in, 2 out]
      }
      event "ON/OFF": Value Change {
        n475 = event-data() -> ()  [unwired: 1 in, 6 out]
        n476 = call <vilib>:"Q.Enqueue Task.vi"("Data1"="ON/OFF", "Task Name"="UUTPower", "Q In"=w988) -> ()  [unwired: 7 in, 2 out]
      }
    }
  }
  "Title" <- "Test Executive" ("Name")
